vi "Lockin_sweep.vi"(0 "Transport":refnum<class "Transport.lvclass">, 3 "error in (no error)":errorcluster) -> (7 "Transport out":refnum<class "Transport.lvclass">, 10 "error out":errorcluster)   [LabVIEW 2019, in "Transport.lvclass"]
uses:
  Transport.lvclass
  Control Experiment/Control Experiment.lvclass
  <userlib>/LevyLab/Lockin-Multichannel/Instrument.DAQ/Typedefs/Sweep.Configuration--Cluster.ctl
  <userlib>/LevyLab/Lockin-Multichannel/Instrument.DAQ/Instrument.DAQ.lvclass
  <userlib>/LevyLab/Lockin-Multichannel/Instrument.DAQ/Typedefs/Sweep.Channel--Cluster.ctl
  <userlib>/LevyLab/Lockin-Multichannel/Instrument.Lockin/Instrument.Lockin.lvclass
  <userlib>/LevyLab/Lockin-Multichannel/Instrument.Lockin/Typedefs/Results Type--Enum.ctl
  <userlib>/LevyLab/Lockin-Multichannel/Instrument.DAQ/Typedefs/Sweep.Pattern--Enum.ctl
  <userlib>/LevyLab/Lockin-Multichannel/Instrument.DAQ/Typedefs/Sweep.Channel--Cluster--Array.ctl
  <vilib>/PRIrvin/XY Utilities/xy_utilities.lvlib
  217905a9-ad64-4e54-8703-31da4ffbd4c0.vi
  9896b5e5-a649-4b1b-acc0-fd49b17a1bc1.vi
  Typedefs/Lockin_Sweep JSON--Cluster.ctl
  <userlib>/LevyLab/Instrument Framework/Instrument Types/Cryostat/Typedefs/Magnet Axis--Enum.ctl
  <userlib>/LevyLab/Instrument Framework/Instrument Types/Cryostat/Instrument.Cryostat.lvclass
  <userlib>/LevyLab/Instrument Framework/Instrument Types/CBridge/Instrument.CBridge.lvclass
  <userlib>/LevyLab/Instrument Framework/Instrument Types/Strain/Instrument.Strain.lvclass
  C:/Program Files/National Instruments/LabVIEW 2019/user.lib/LevyLab/Instrument Framework/Instrument/Instrument.lvclass
  C:/Program Files/National Instruments/LabVIEW 2019/vi.lib/JKI/JKI SMO/SMO/SMO.lvclass
  <vilib>/PRIrvin/XY Utilities/subVIs/Divide float (multiple).vi
  <vilib>/PRIrvin/XY Utilities/subVIs/Multiply float (multiple).vi
  <vilib>/Utility/Data Type/NI_Data Type.lvlib
  <userlib>/LevyLab/Instrument Framework/Instrument/Instrument.lvclass
  <userlib>/LevyLab/Instrument Framework/Instrument Types/Lockin/Instrument.LockinAPI.lvclass
  <userlib>/LevyLab/Instrument Framework/Instrument Types/Amplifier/Instrument.Amplifier.lvclass
  <userlib>/LevyLab/Instrument Framework/Instrument Types/Delay Line/Instrument.DelayLine.lvclass
  <userlib>/LevyLab/Instrument Framework/Instrument Types/VNA/Instrument.VNA.lvclass
  <userlib>/LevyLab/Instrument Framework/Instrument Types/VSource/Instrument.VSource.lvclass
  Control Experiment/Typedefs/Instrument Types--enum.ctl
  Attributes/Instrument Attributes.lvlib
  ac72d6f7-f5c3-431a-8621-5120436d0f52.vi
  C:/Program Files/National Instruments/LabVIEW 2019/user.lib/LevyLab/Instrument Framework/Instrument Types/Lockin/Instrument.LockinAPI.lvclass
panel:
  in  "Start":bool
  in  "stop":bool
  in  "Tab Control":T1(tab)
  out "state history":string
  in  "Sweep Tables":cluster{"Ch":i32, "Table":dbl[]}[](array[cluster]) {"Table" format="%#_3p"; "Ch" min=1 max=16}
  in  "Emergency Stop Visible?":bool
  out "elapsed time (s)":i32=231
  in  "Experiment Comments":string
  in  "Experiment Folder":string
  out "time b/w points (ms)":u32=1037
  in  "Sweep Channels":T2 {"Table" format="%#_1f"; "Channel" min=1 max=128; "Start" format="%#_6p"; "End" format="%#_6p"}
  in  "Sweep Time (s)":dbl
  in  "Initial Wait (s)":dbl
  in  "Return to Start":bool
  out "Instrument Status":string
  in  "Emergency Stop 1":bool caption="Emergency Stop"
  out "Lockin (X)":cluster{"Wavenumber":dbl[], "Data":dbl[]}[](graph)
  out "Lockin (Y)":cluster{"Wavenumber":dbl[], "Data":dbl[]}[](graph)
  in  "Units":enum16{"ohms & siemens", "h/e2 & e2/h"}(ring)
  out "Resistance":cluster{"X-array":dbl[], "Y-array":dbl[]}[](graph)
  out "Conductance":cluster{"X-array":dbl[], "Y-array":dbl[]}[](graph)
  in  "Emergency Stop 2":bool caption="Emergency Stop"
  out "AI":cluster{"Wavenumber":dbl[], "Data":dbl[]}[](graph)
  out "AO":cluster{"Wavenumber":dbl[], "Data":dbl[]}[](graph)
  in  "Emergency Stop 3":bool caption="Emergency Stop"
  out "2 Terminal":cluster{"Wavenumber":dbl[], "Data":dbl[]}[](graph)
  out "4 Terminal":cluster{"Wavenumber":dbl[], "Data":dbl[]}[](graph)
  in  "Emergency Stop 4":bool caption="Emergency Stop"
  # "Configuration"
  # "Status"
  # "Metadata"
  # "VI Description"
  # "This VI uses the Lockin Sweep Method. That is, you tell the lockin to sweep from Start to End in a certain amount of time. The lockin will run independently while it executes the sweep. While the lockin is sweeping, this VI will poll the lockin once per second to get a snapshot of current results and the sweep status (sweeping or not sweeping). When the lockin is finished sweeping this VI will ask for the final sweep results and save them. The spacing between points is determined by the \"Fs Output\" control in the Lockin."
  # "*** These controls are only read if this VI is the top level. If is is called from Sweep Control then the folder and comments come from Sweep Control.vi ***"
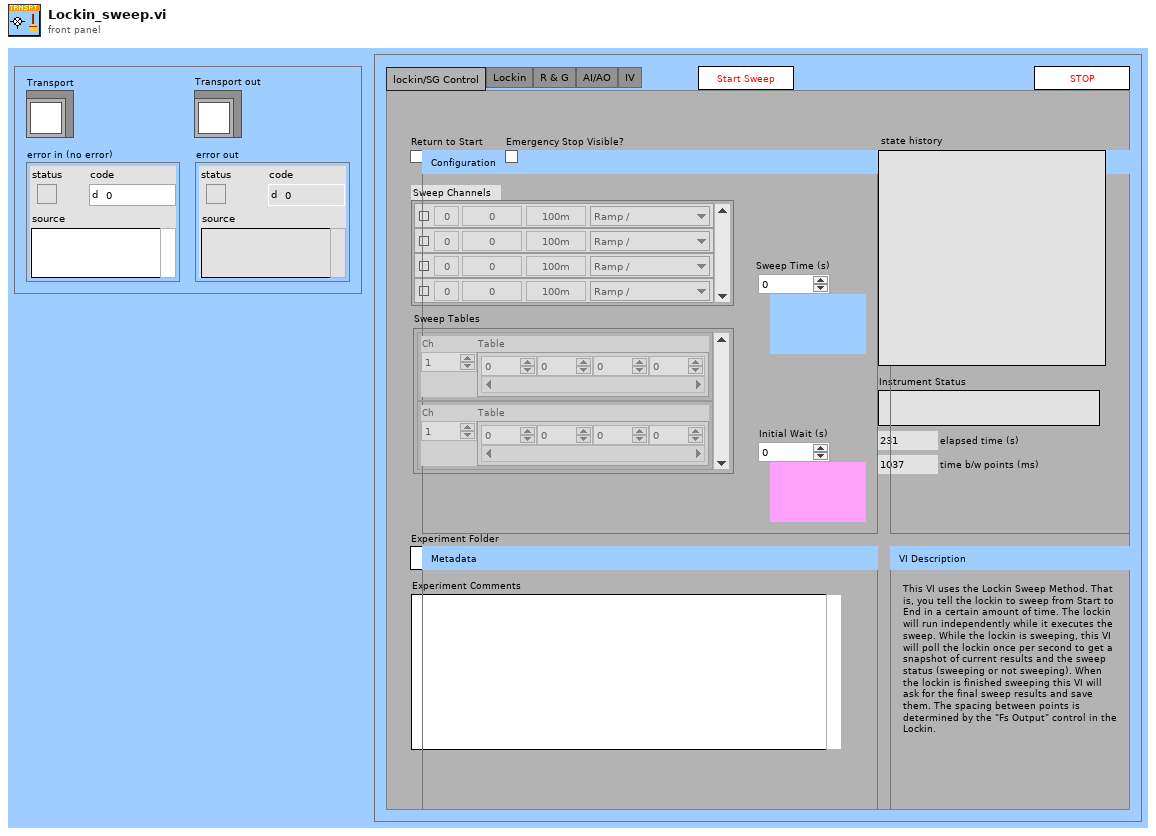
[diagram p1: front panel]
types:
  T1 = enum32{"lockin/SG Control", "Lockin", "R & G", "AI/AO", "IV"}
  T2 = typedef "Instrument.Lockin.lvlib/Instrument.DAQ.lvclass/Sweep.Channel--Cluster--Array.ctl" = T3[]
  T3 = typedef "Instrument.Lockin.lvlib/Instrument.DAQ.lvclass/Sweep.Channel--Cluster.ctl" = cluster{"Enable?":bool, "Channel":u16, "Start":dbl, "End":dbl, "Pattern":T4, "Table":dbl[]}
  T4 = typedef "Instrument.Lockin.lvlib/Instrument.DAQ.lvclass/Sweep.Pattern--Enum.ctl" = enum16{"Ramp /", "Ramp /\\", "Smooth Ramp _/", "Smooth Ramp _/\\_", "Table"}
  T5 = enum32{"Invalid", "Standard", "Closed", "Hidden", "Minimized", "Maximized"}
  T6 = enum32{"invalid app kind", "Development System", "Run Time System", "Student Edition", "Embedded LabVIEW", "Evaluation", "Custom"}
  T7 = enum32{"Bad", "Idle", "Run top level", "Running"}
  T8 = typedef "Control Experiment.lvclass/Instrument Types--enum.ctl" = enum16{"DAQ", "Amplifier", "Temperature", "Magnet", "Rotator", "Level", "Capacitance", "Delay Line", "Strain Cell", "VNA", "Source"}
  T9 = typedef "Instrument.Lockin.lvlib/Instrument.Lockin.lvclass/Results Type--Enum.ctl" = enum16{"X", "Y", "R", "Theta", "Mean"}
  T10 = typedef "Instrument.Lockin.lvlib/Instrument.DAQ.lvclass/Sweep.Configuration--Cluster.ctl" = cluster{"Sweep Time (s)":dbl, "Initial Wait (s)":dbl, "Return to Start":bool, "Channels":T2}
  T11 = typedef "Instrument.Cryostat.lvclass/Magnet Axis--Enum.ctl" = enum16{"X", "Y", "Z"}
  T12 = typedef "Transport.lvclass/Lockin_Sweep JSON--Cluster.ctl" = cluster{"Sweep Time (s)":dbl, "Initial Wait (s)":dbl, "Return to Start":bool, "Sweep Channels":T2, "Sweep Tables":cluster{"Ch":i32, "Table":dbl[]}[]}
  T13 = typedef "Control Experiment.lvclass/Instrument Classes--cluster.ctl" = cluster{"DAQ":refnum<class "Instrument.LockinAPI.lvclass">, "Amplifier":refnum<class "Instrument.Amplifier.lvclass">, "Temperature":refnum<class "Instrument.Cryostat.lvclass">, "Magnet":refnum<class "Instrument.Cryostat.lvclass">, "Rotator":refnum<class "Instrument.Cryostat.lvclass">, "Level":refnum<class "Instrument.Cryostat.lvclass">, "Capacitance":refnum<class "Instrument.CBridge.lvclass">, "Delay Line":refnum<class "Instrument.DelayLine.lvclass">, "Strain Cell":refnum<class "Instrument.Strain.lvclass">, "VNA":refnum<class "Instrument.VNA.lvclass">, "Source":refnum<class "Instrument.VSource.lvclass">}
  T14 = cluster{"Core":cluster{"Current VI Reference":refnum<vi>, "Close Panel on Exit?":bool}, "Transport":refnum<class "Transport.lvclass">, "C.E.":refnum<class "Control Experiment.lvclass">, "Instruments":T13, "Time":dbl, "Temperature":dbl, "Magnet":dbl, "Results (Dictionary)":cluster{"key":string, "value":dbl}[], "Sweep Value":dbl, "ms [0]":u32, "ms [i]":u32, "Execution:State":enum32{"Bad", "Idle", "Run top level", "Running"}, "Run Time System?":bool, "AO Waveforrm":waveform(dbl)[], "AI Waveform":waveform(dbl)[], "Sweep_AO":waveform(dbl)[], "Sweep_AI":waveform(dbl)[], "Sweep_X":waveform(dbl)[], "Sweep_Y":waveform(dbl)[], "Amplitude":dbl[], "UI stop":bool}
  T15 = cluster{"Current VI Reference":refnum<vi>, "Close Panel on Exit?":bool}
  T16 = cluster{"I-":i32, "I+":i32, "V1-":i32, "V1+":i32, "I2-":i32, "I2+":i32, "V2-":i32, "V2+":i32}
  T17 = typedef "Instrument.LockinAPI.lvclass/LockinAPI.getState.states--enum.ctl" = enum16{"idle", "created", "started", "stopped", "sweeping"}
  T18 = typedef "Instrument.Lockin.lvlib/Instrument.DAQ.lvclass/AO.Channel--Cluster--Array.ctl" = T19[]
  T19 = typedef "Instrument.Lockin.lvlib/Instrument.DAQ.lvclass/AO.Channel--Cluster.ctl" = cluster{"Enable?":bool, "Channel":i32, "Amplitude":dbl, "Offset":dbl, "Frequency":dbl, "Phase":dbl, "Function":T20, "Sweeping?":bool, "Limit AC":bool, "Limit DC?":bool, "Duty Cycle":bool}
  T20 = typedef "Instrument.Lockin.lvlib/Instrument.DAQ.lvclass/AO.Channel.Function--Enum.ctl" = enum16{"sine", "square", "triangle", "saw"}
  T21 = typedef "Instrument.LockinAPI.lvclass/LockinAPI.SweepData--Cluster.ctl" = cluster{"AO":waveform(dbl)[], "AI":waveform(dbl)[], "X":waveform(dbl)[], "Y":waveform(dbl)[]}
  T22 = typedef "LV-Data.lvclass/Dictionary--cluster.ctl" = cluster{"key":string, "value":variant}
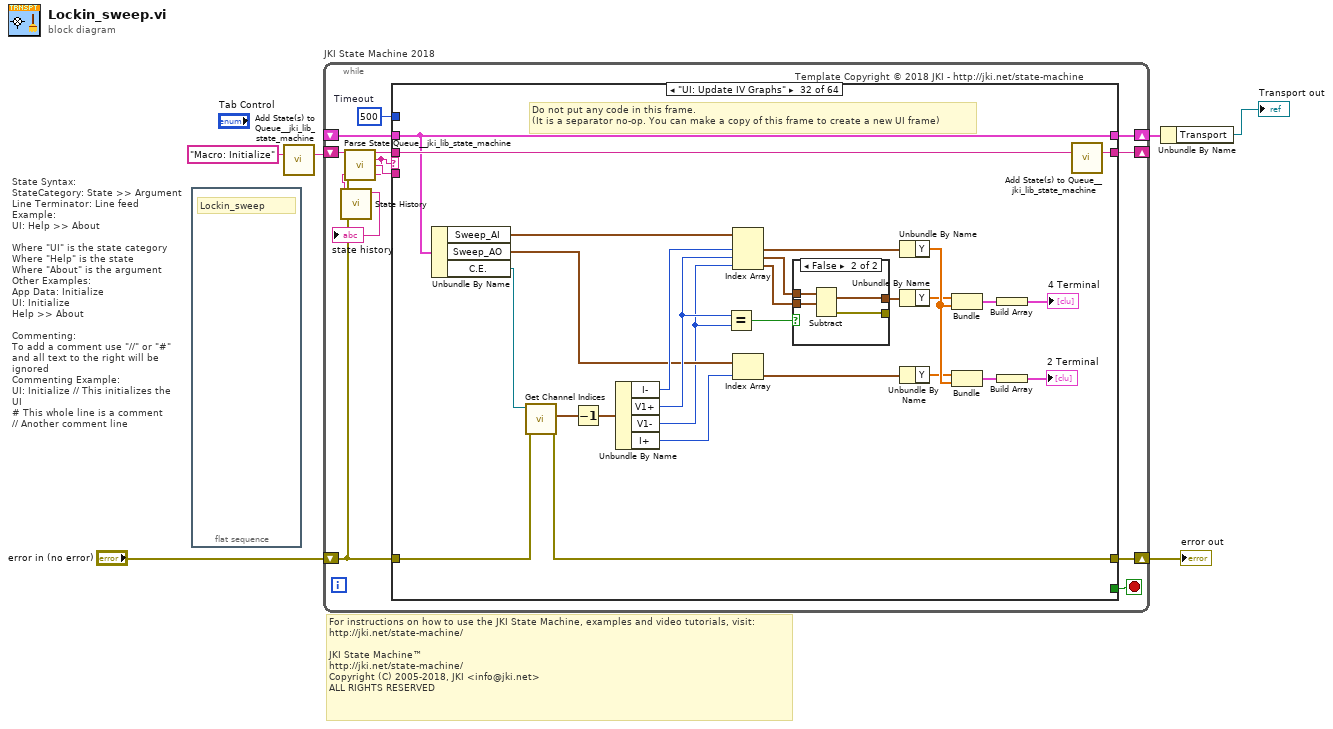
[diagram p0: block diagram]
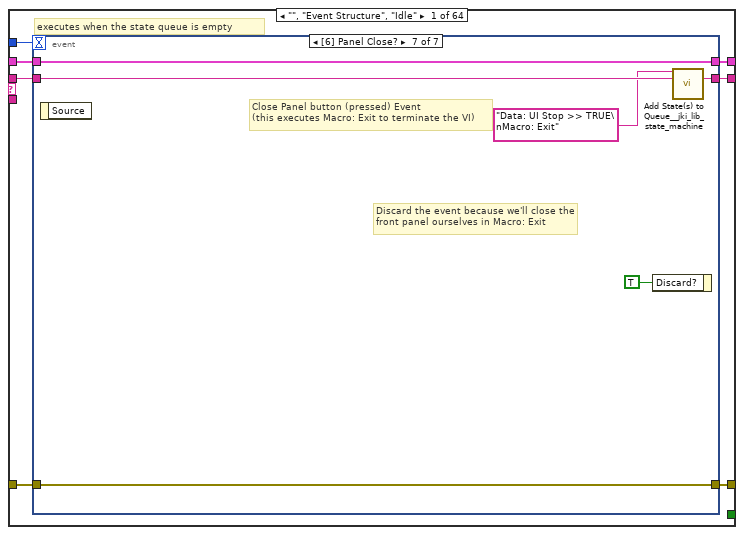
[diagram p2: hidden frame]
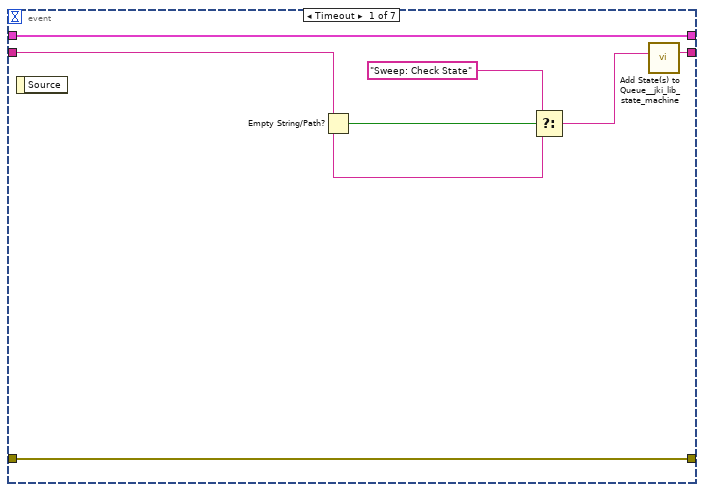
[diagram p3: hidden frame]
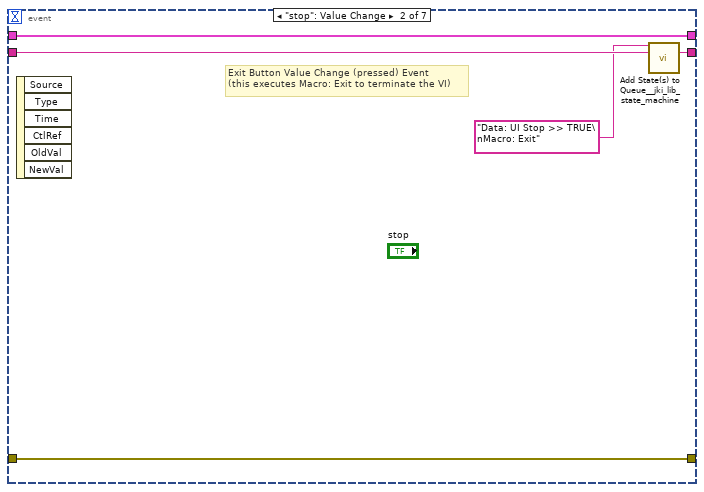
[diagram p4: hidden frame]
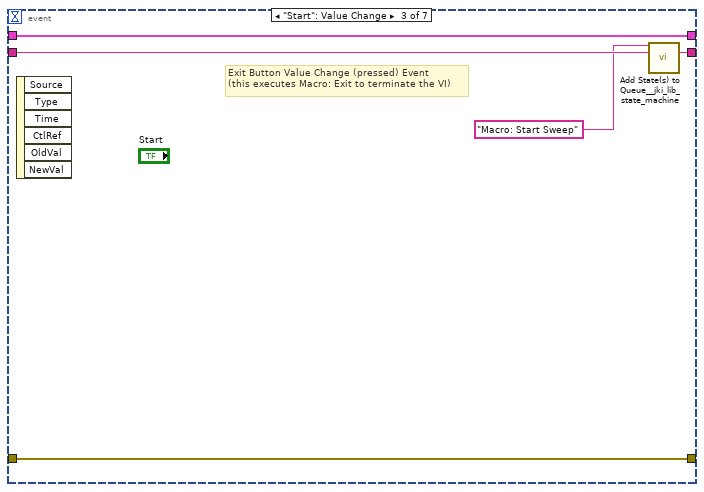
[diagram p5: hidden frame]
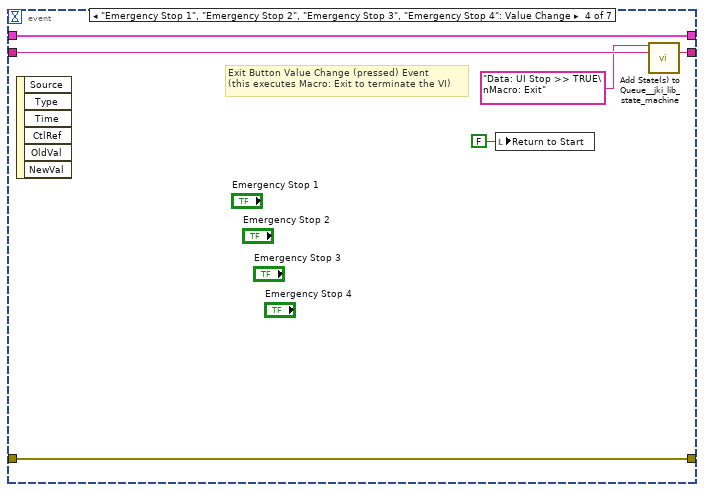
[diagram p6: hidden frame]
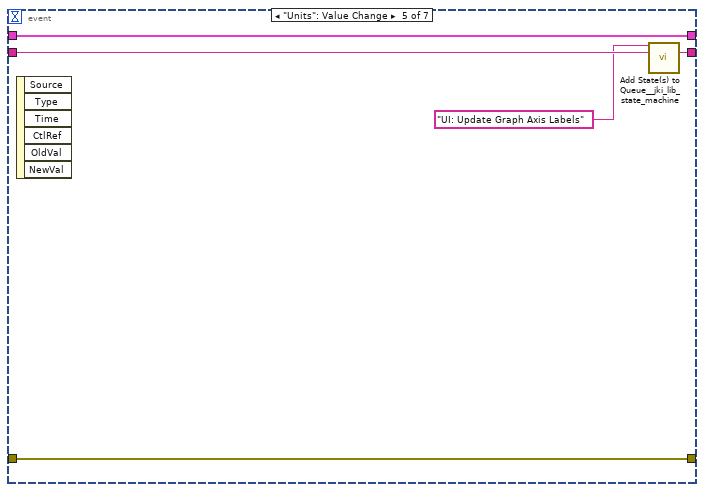
[diagram p7: hidden frame]
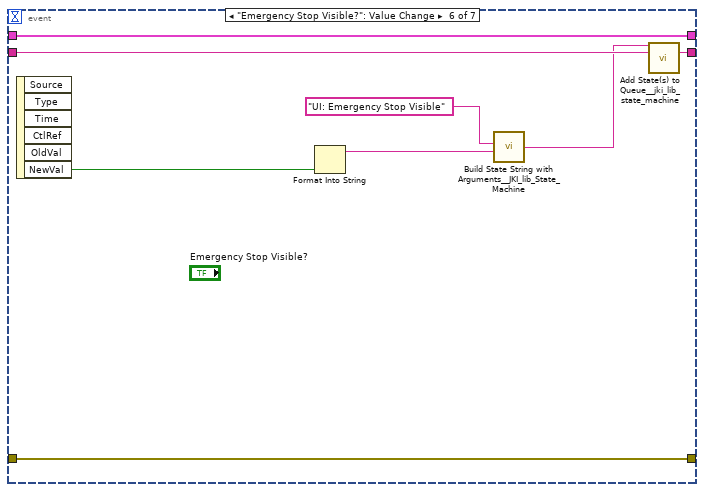
[diagram p8: hidden frame]
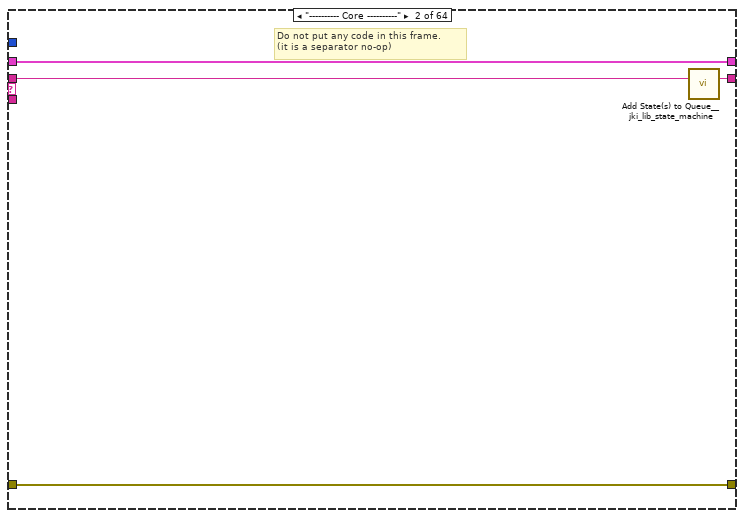
[diagram p9: hidden frame]
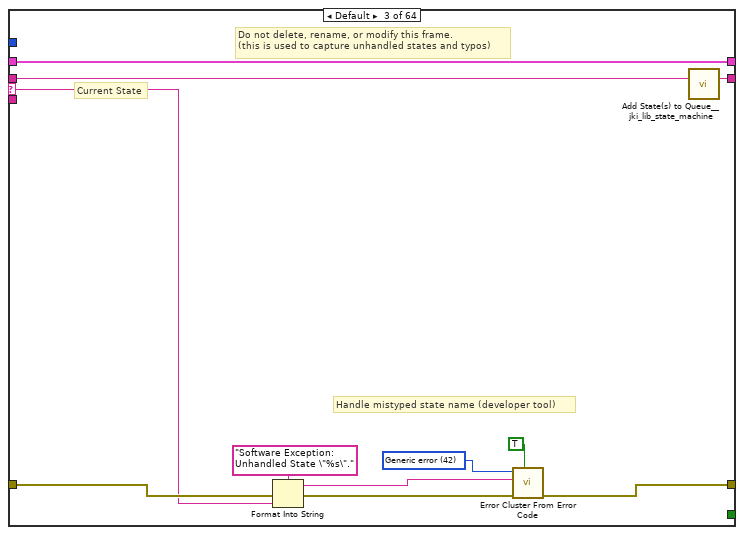
[diagram p10: hidden frame]
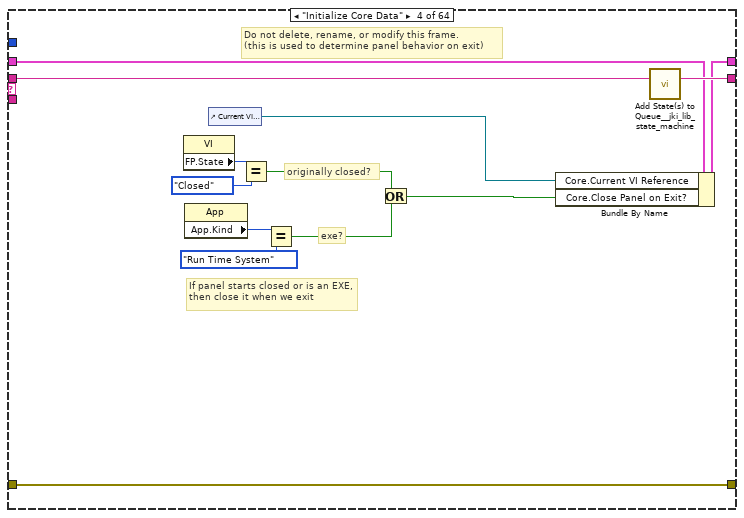
[diagram p11: hidden frame]
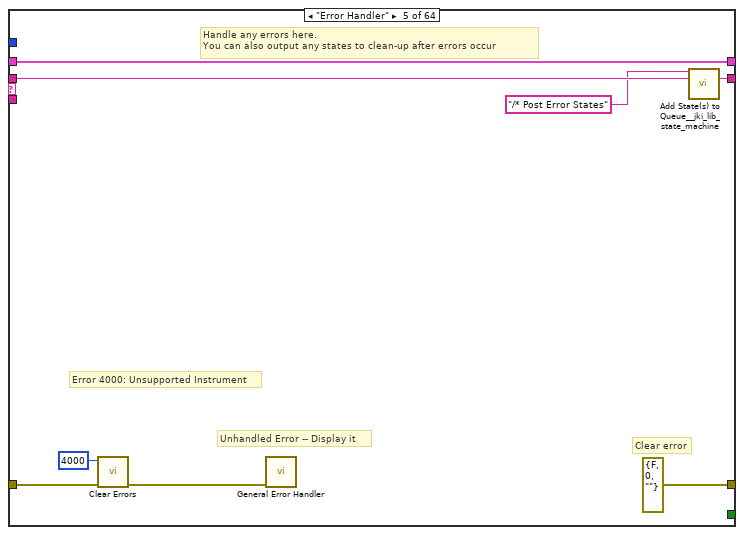
[diagram p12: hidden frame]
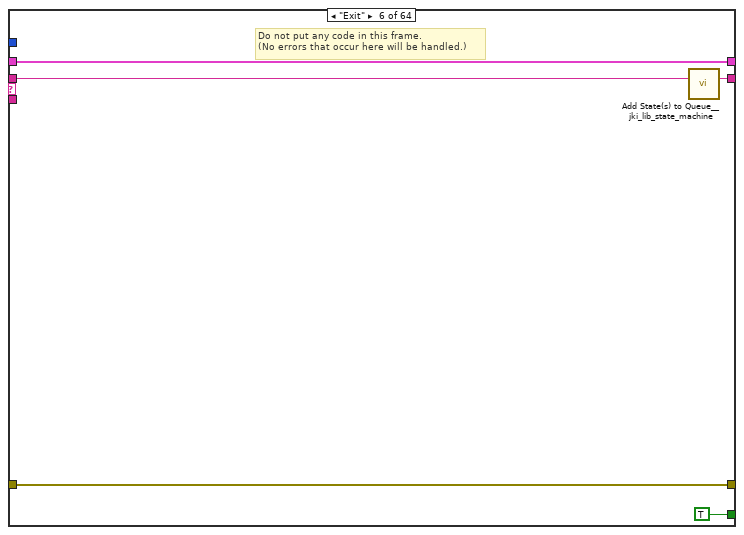
[diagram p13: hidden frame]
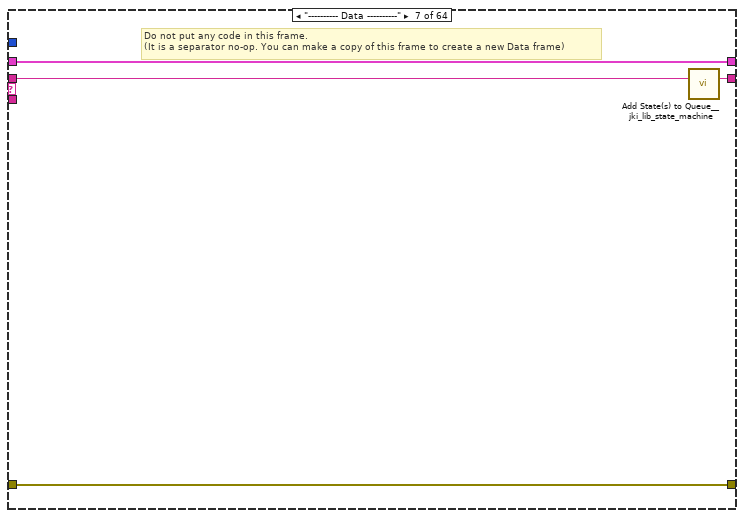
[diagram p14: hidden frame]
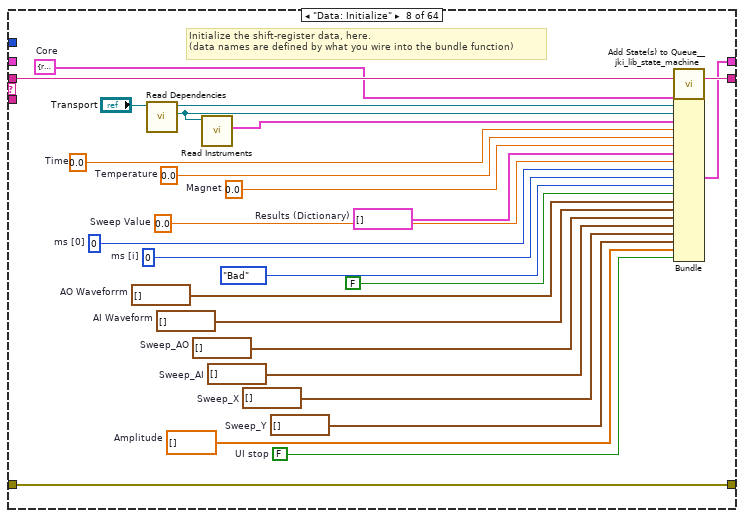
[diagram p15: hidden frame]
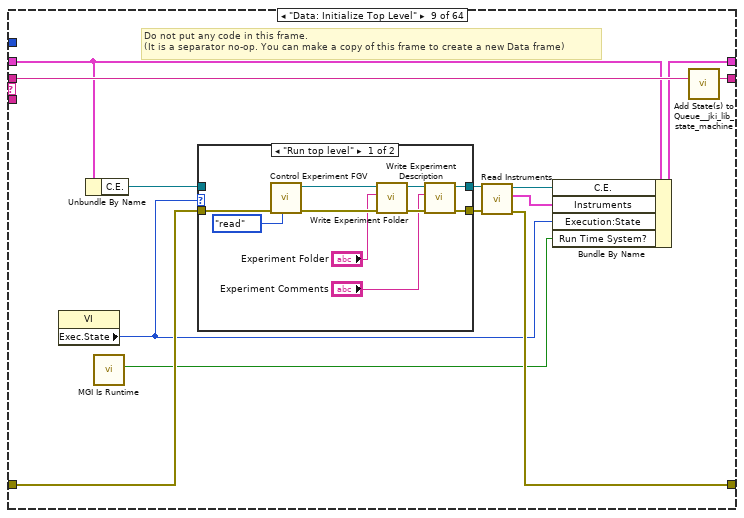
[diagram p16: hidden frame]
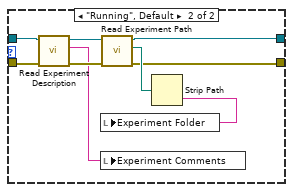
[diagram p17: hidden frame]
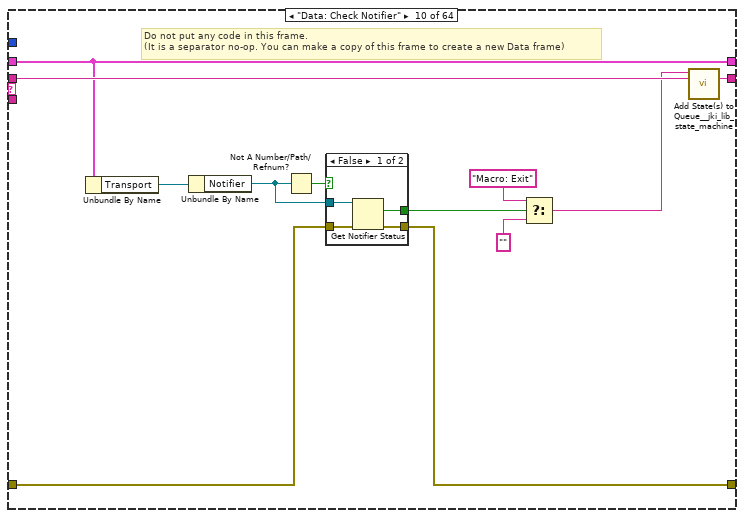
[diagram p18: hidden frame]
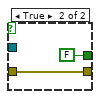
[diagram p19: hidden frame]
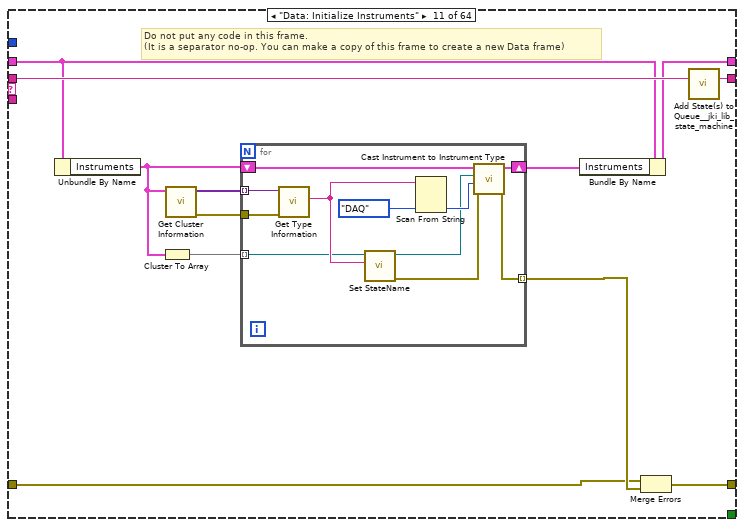
[diagram p20: hidden frame]
diagram:
  # "For instructions on how to use the JKI State Machine, examples and video tutorials, visit:\nhttp://jki.net/state-machine/\n\nJKI State Machine™\nhttp://jki.net/state-machine/\nCopyright (C) 2005-2018, JKI <info@jki.net>\nALL RIGHTS RESERVED"
  # "State Syntax:\nStateCategory: State >> Argument\nLine Terminator: Line feed\nExample:\nUI: Help >> About\n\nWhere \"UI\" is the state category\nWhere \"Help\" is the state\nWhere \"About\" is the argument\nOther Examples:\nApp Data: Initialize\nUI: Initialize\nHelp >> About\n\nCommenting:\nTo add a comment use \"//\" or \"#\" and all text to the right will be ignored\nCommenting Example:\nUI: Initialize // This initializes the UI\n# This whole line is a comment\n// Another comment line"
  n1 = flat-sequence {
    frame #0 {
      # "Lockin_sweep"
    }
  }
  n2 = call <vilib>:"Add State(s) to Queue__jki_lib_state_machine.vi"("State(s) in (\"\")"="Macro: Initialize") -> ("States Out"=w6:string)  [unwired: 14 in]
  n3 = while "JKI State Machine 2018" {
    shift-right: [w13] -> w4
    shift-left: _ -> [w12]
    shift-right: [w16] -> w2
    shift-left: "error in (no error)" -> [w10]
    shift-right: [w15] -> _
    shift-left: w6 -> [w9]
    stop <- w14 stop-if-true
    w11 = 500  # Timeout
    # "Template Copyright © 2018 JKI - http://jki.net/state-machine"
    n4 = call <vilib>:"Parse State Queue__jki_lib_state_machine.vi"("State Queue"=w9, "Error In (no error)"=w10) -> ("Remaining States"=w18:string, "Current State"=w8:string, "Arguments"=w17:string)  [unwired: 11 in]
    n5 = call "State History.vi"("Current State"=w8) -> ("History"=→"state history":string)  [unwired: 10 in]
    n6 = case shown="\"UI: Update IV Graphs\"" w8 {
      selector: w8 -> [_ _ w72 _ _ _ _ _ _ _ _ _ _ _ _ _ _ _ _ _ _ _ _ _ _ _ _ _ _ _ _ _ _ _ _ _ _ _ _ _ _ _ _ _ _ _ _ _ _ _ _ _ _ _ _ _ _ _ _ _ _ _ _ _]
      tunnel: w18 -> [w25 w71 w76 w95 w103 w108 w112 w138 w151 w182 w200 w224 w255 w290 w302 w329 w347 w359 w370 w376 w387 w403 w418 w444 w461 w481 w519 w568 w593 w608 w626 w673 w685 w754 w764 w769 w782 w795 w800 w812 w823 w827 w860 w886 w898 w912 w936 w949 w953 w957 w968 w983 w1005 w1033 w1066 w1088 w1110 w1132 w1164 w1185 w1189 w1193 w1213 w1232]
      tunnel: w17 -> [_ _ _ _ _ _ _ _ _ _ _ _ _ _ _ w324 _ _ _ w371 w383 _ w405 _ _ _ _ w562 w582 _ _ _ w679 _ _ _ _ _ _ _ _ _ _ _ _ _ _ _ _ _ _ _ _ _ _ _ _ _ _ _ _ _ _ _]
      tunnel: w12 -> [w23 w68 w74 w88 w100 w106 w109 _ w141 w180 w197 w221 w252 w275 w296 w325 w339 w356 w361 w374 w384 w399 w415 w434 w457 w478 w516 w566 w585 w600 w623 w663 w681 w751 w757 w766 w778 w791 w796 w804 w820 w824 w857 w884 w892 w910 w934 w946 w951 w954 w961 w977 w998 w1024 w1060 w1082 w1104 w1126 w1156 w1183 w1186 w1190 w1201 w1227]
      tunnel: [w22 w69 w78 w92 errorcluster {"status"=FALSE, "code"=0, "source"=""} ("error out") w105 w110 w135 w143 w173 w196 w214 w251 w277 w294 w327 w340 w357 w363 w372 w385 w395 w416 w439 w459 w479 w517 w565 w586 w606 w624 w654 w682 w752 w762 w767 w771 w793 w798 w810 w821 w825 w828 w879 w896 w905 w923 w947 w950 w955 w959 w971 w993 w1022 w1053 w1076 w1098 w1120 w1162 w1180 w1187 w1191 w1204 w1225] -> w16
      tunnel: w10 -> [w21 w69 w77 w92 w97 w105 w110 w135 w144 w172 w189 w215 w250 w284 w297 w327 w331 w357 w368 w373 w385 w390 w416 w438 w455 w470 w503 w565 w580 w606 w624 w655 w683 w752 w762 w767 w770 w793 w798 w810 w821 w825 w834 w875 w887 w901 w913 w947 w950 w955 w960 w981 w1000 w1020 w1061 w1083 w1105 w1127 w1140 w1171 w1187 w1191 w1196 w1220]
      tunnel: [w24 w70 w75 w94 w102 w107 w111 w137 w150 w181 w199 w223 w254 w289 w301 w328 w346 w358 w369 w375 w386 w402 w417 w443 w460 w480 w518 w567 w592 w607 w625 w672 w684 w753 w763 w768 w781 w794 w799 w811 w822 w826 w859 w885 w897 w911 w935 w948 w952 w956 w967 w982 w1004 w1032 w1065 w1087 w1109 w1131 w1163 w1184 w1188 w1192 w1212 w1231] -> w15
      tunnel: [_ _ _ _ _ TRUE _ _ _ _ _ _ _ _ _ _ _ _ _ _ _ _ _ _ _ _ _ _ _ _ _ _ _ _ _ _ _ _ _ _ _ _ _ _ _ _ _ _ _ _ _ _ _ _ _ _ _ _ _ _ _ _ _ _] -> w14
      tunnel: [w20 w68 w74 w93 w100 w106 w109 w136 w142 w180 w198 w222 w253 w285 w295 w326 w343 w356 w364 w374 w384 w398 w415 w434 w457 w478 w516 w566 w585 w600 w623 w663 w681 w751 w757 w766 w778 w791 w796 w804 w820 w824 w858 w883 w893 w909 w933 w946 w951 w954 w965 w980 w1003 w1025 w1064 w1086 w1108 w1130 w1155 w1182 w1186 w1190 w1202 w1228] -> w13
      tunnel: w11 -> [w19 _ _ _ _ _ _ _ _ _ _ _ _ _ _ _ _ _ _ _ _ _ _ _ _ _ _ _ _ _ _ _ _ _ _ _ _ _ _ _ _ _ _ _ _ _ _ _ _ _ _ _ _ _ _ _ _ _ _ _ _ _ _ _]
      frame "", "Event Structure", "Idle" {
        # "executes when the state queue is empty"
        n7 = event shown="[6] Panel Close?" {
          selector: _ -> [_ _ _ _ _ _ _]
          dyn-events: _ -> [_ _ _ _ _ _ _]
          timeout: w19 -> [_ _ _ _ _ _ _]
          tunnel: w25 -> [w27 w37 w42 w48 w53 w61 w67]
          tunnel: [w32 w36 w41 w47 w52 w60 w66] -> w24
          tunnel: w23 -> [w30 w33 w38 w45 w50 w58 w64]
          tunnel: [w31 w35 w40 w46 w51 w59 w65] -> w22
          tunnel: w21 -> [w31 w35 w40 w46 w51 w59 w65]
          tunnel: [w30 w33 w38 w45 w50 w58 w64] -> w20
          event Timeout {
            n8 = event-data() -> ()  [unwired: 1 in, 1 out]
            n9 = Empty String/Path?(string/path=w27) -> (empty?=w29:bool)
            n10 = Select(t="Sweep: Check State" ("State(s) in Front (\"\")"), s=w29, f=w27) -> (s? t:f=w28:string)
            n11 = call <vilib>:"Add State(s) to Queue__jki_lib_state_machine.vi"("State(s) in (\"\")"=w28) -> ("States Out"=w32:string)  [unwired: 14 in]
          }
          event "stop": Value Change {
            # "Exit Button Value Change (pressed) Event\n(this executes Macro: Exit to terminate the VI)"
            n12 = event-data() -> ()  [unwired: 1 in, 6 out]
            n13 = call <vilib>:"Add State(s) to Queue__jki_lib_state_machine.vi"("State(s) in Front (\"\")"="Data: UI Stop >> TRUE\nMacro: Exit", "State(s) in (\"\")"=w37) -> ("States Out"=w36:string)  [unwired: 13 in]
          }
          event "Start": Value Change {
            # "Exit Button Value Change (pressed) Event\n(this executes Macro: Exit to terminate the VI)"
            n14 = event-data() -> ()  [unwired: 1 in, 6 out]
            n15 = call <vilib>:"Add State(s) to Queue__jki_lib_state_machine.vi"("State(s) in Front (\"\")"="Macro: Start Sweep", "State(s) in (\"\")"=w42) -> ("States Out"=w41:string)  [unwired: 13 in]
          }
          event "Emergency Stop 1", "Emergency Stop 2", "Emergency Stop 3", "Emergency Stop 4": Value Change {
            # "Exit Button Value Change (pressed) Event\n(this executes Macro: Exit to terminate the VI)"
            n16 = event-data() -> ()  [unwired: 1 in, 6 out]
            n17 = local write "Return to Start"(FALSE ("Return to Start")) -> ()
            n18 = call <vilib>:"Add State(s) to Queue__jki_lib_state_machine.vi"("State(s) in Front (\"\")"="Data: UI Stop >> TRUE\nMacro: Exit", "State(s) in (\"\")"=w48) -> ("States Out"=w47:string)  [unwired: 13 in]
          }
          event "Units": Value Change {
            n19 = event-data() -> ()  [unwired: 1 in, 6 out]
            n20 = call <vilib>:"Add State(s) to Queue__jki_lib_state_machine.vi"("State(s) in Front (\"\")"="UI: Update Graph Axis Labels", "State(s) in (\"\")"=w53) -> ("States Out"=w52:string)  [unwired: 13 in]
          }
          event "Emergency Stop Visible?": Value Change {
            n21 = event-data() -> ("NewVal"=w55:bool)  [unwired: 1 in, 5 out]
            n22 = Format Into String(w55) -> (resulting string=w57:string)  [unwired: 3 in, 1 out]
            n23 = call <vilib>:"Build State String with Arguments__JKI_lib_State_Machine.vi"("Arguments (\"\")"=w57, "State"="UI: Emergency Stop Visible") -> ("State with Arguments"=w54:string)  [unwired: 4 in]
            n24 = call <vilib>:"Add State(s) to Queue__jki_lib_state_machine.vi"("State(s) in Front (\"\")"=w54, "State(s) in (\"\")"=w61) -> ("States Out"=w60:string)  [unwired: 13 in]
          }
          event Panel Close? {
            # "Discard the event because we'll close the front panel ourselves in Macro: Exit"
            # "Close Panel button (pressed) Event\n(this executes Macro: Exit to terminate the VI)"
            n25 = event-data() -> ()  [unwired: 1 in, 1 out]
            n26 = event-data("Discard?"=TRUE) -> ()  [unwired: 1 in, 1 out]
            n27 = call <vilib>:"Add State(s) to Queue__jki_lib_state_machine.vi"("State(s) in Front (\"\")"="Data: UI Stop >> TRUE\nMacro: Exit", "State(s) in (\"\")"=w67) -> ("States Out"=w66:string)  [unwired: 13 in]
          }
        }
      }
      frame "---------- Core ----------" {
        # "Do not put any code in this frame.\n(it is a separator no-op)"
        n28 = call <vilib>:"Add State(s) to Queue__jki_lib_state_machine.vi"("State(s) in (\"\")"=w71) -> ("States Out"=w70:string)  [unwired: 14 in]
      }
      frame Default {
        w81 = 42 items=["No error", "Argument error", "Memory is full", "Out of zone", "End of file", "File already open", "Generic file I/O error", "File not found", "File permission error", "Disk is full", "Duplicate path", "Too many files open", "System feature not enabled", "Resource file not found", "Cannot add resource", "Resource not found", "Image not found", "Image memory error", "Pen does not exist", "Config type invalid", "Config token not found", "Config parse error", "Config memory error", "Bad external code format", "Bad external code offset", "External code not present", "Null window", "Destroy window error", "Null menu", "Print aborted", "Bad print record", "Print driver error", "Windows error during printing", "Memory error during printing", "Print dialog error", "Generic print error", "Invalid device refnum", "Device not found", "Device parameter error", "Device unit error", "Cannot open device", "Device call aborted", "Generic error", "Cancelled by user", "Object ID too low", "Object ID too high", "Object not in heap", "Unknown heap", "Unknown object (invalid DefProc)", "Unknown object (DefProc not in table)", "Message out of range", "Invalid (null) method", "Unknown message", "Manager call not supported", "Bad address", "Network operation in progress", "Network operation timed out", "Connection is busy", "Network attribute not supported", "Network error", "Address in use", "System out of memory", "Connection aborted", "Connection refused", "Not connected", "Already connected", "Connection closed", "Initialization error (interapplication manager)", "Bad occurrence", "Wait on unbound occurrence handler", "Occurrence queue overflow", "Datalog type conflict", "Unused", "Unrecognized type (interapplication manager)", "Memory corrupt", "Failed to make temporary DLL", "Old CIN version", "Drag socket not found", "Failed to load drop-object", "Failed to register OLE object", "Failed to release OLE object", "Format specifier type mismatch", "Unknown format specifier", "Too few format specifiers", "Too many format specifiers", "Scan failed", "Newer CIN version", "Error converting to variant", "Runtime menu error", "Password tampered", "Variant attribute not found", "Incompatible variant data type", "Event data is not available", "Event Store is not present", "Occurrence is not found", "Event Queue is not created", "Event info is not available", "Refnum passed is NULL", "Error retrieving Class GUID", "Error retrieving CoClass GUID", "Error retrieving TypeLib GUID.", "Bad built application magic bytes.", "Specific driver is different from the specific driver associated with the Logical Name.", "There is no session opened to the class driver.", "Max Error", "MAX - Error with config objects", "MAX - Error loading configuration", "MAX - Group not supported"]
        # "Current State"
        # "Do not delete, rename, or modify this frame.\n(this is used to capture unhandled states and typos)"
        # "Handle mistyped state name (developer tool)"
        n29 = Format Into String(format string="Software Exception: Unhandled State \"%s\"." ("message"), error in=w77, w72) -> (resulting string=w80:string, error out=w79:errorcluster)  [unwired: 1 in]
        n30 = call <vilib>:"Error Cluster From Error Code.vi"("show call chain? (False)"=TRUE, "error in (no error)"=w79, "error message (\"\")"=w80, "error code (0)"=w81) -> ("error out"=w78:errorcluster)  [unwired: 5 in]
        n31 = call <vilib>:"Add State(s) to Queue__jki_lib_state_machine.vi"("State(s) in (\"\")"=w76) -> ("States Out"=w75:string)  [unwired: 14 in]
      }
      frame "Initialize Core Data" {
        # "Do not delete, rename, or modify this frame.\n(this is used to determine panel behavior on exit)"
        # "originally closed?"
        # "exe?"
        # "If panel starts closed or is an EXE, then close it when we exit"
        n32 = property class="VI"() -> ("FP.State"=w85:T5)  [unwired: 2 in, 2 out]
        n33 = property class="App"() -> ("App.Kind"=w91:T6)  [unwired: 2 in, 2 out]
        n34 = control-ref of="Current VI Reference"() -> (w86:refnum<vi>)
        n35 = Equal?(x=w85, y=T5."Closed" ("Front Panel Window:State")) -> (x = y?=w83:bool)
        n36 = Equal?(x=w91, y=T6."Run Time System" ("Application:Kind")) -> (x = y?=w89:bool)
        n37 = Or(x=w83, y=w89) -> (x .or. y?=w87:bool)
        n38 = Bundle By Name(cluster=w88, "Core.Current VI Reference"=w86, "Core.Close Panel on Exit?"=w87) -> (w93:T14)
        n39 = call <vilib>:"Add State(s) to Queue__jki_lib_state_machine.vi"("State(s) in (\"\")"=w95) -> ("States Out"=w94:string)  [unwired: 14 in]
      }
      frame "Error Handler" {
        # "Error 4000: Unsupported Instrument"
        # "Unhandled Error -- Display it"
        # "Handle any errors here.\nYou can also output any states to clean-up after errors occur"
        # "Clear error"
        n40 = call <vilib>:"Clear Errors.vi"("error in (no error)"=w97, "specific error code to clear (0: all)"=4000) -> ("error out"=w96:errorcluster)  [unwired: 4 in, 1 out]
        n41 = call <vilib>:"General Error Handler.vi"("error in (no error)"=w96) -> ()  [unwired: 10 in, 5 out]
        n42 = call <vilib>:"Add State(s) to Queue__jki_lib_state_machine.vi"("State(s) in Front (\"\")"="/* Post Error States", "State(s) in (\"\")"=w103) -> ("States Out"=w102:string)  [unwired: 13 in]
      }
      frame "Exit" {
        # "Do not put any code in this frame.\n(No errors that occur here will be handled.)"
        n43 = call <vilib>:"Add State(s) to Queue__jki_lib_state_machine.vi"("State(s) in (\"\")"=w108) -> ("States Out"=w107:string)  [unwired: 14 in]
      }
      frame "---------- Data ----------" {
        # "Do not put any code in this frame.\n(It is a separator no-op. You can make a copy of this frame to create a new Data frame)"
        n44 = call <vilib>:"Add State(s) to Queue__jki_lib_state_machine.vi"("State(s) in (\"\")"=w112) -> ("States Out"=w111:string)  [unwired: 14 in]
      }
      frame "Data: Initialize" {
        w115 = FALSE  # UI stop
        w118 = dbl[] []  # Amplitude
        w122 = waveform(dbl)[] []  # Sweep_Y
        w123 = waveform(dbl)[] []  # Sweep_X
        w119 = cluster{"key":string, "value":dbl}[] []  # Results (Dictionary)
        w125 = waveform(dbl)[] []  # Sweep_AO
        w124 = waveform(dbl)[] []  # Sweep_AI
        w126 = waveform(dbl)[] []  # AI Waveform
        w127 = waveform(dbl)[] []  # AO Waveforrm
        w128 = 0.0  # Sweep Value
        w129 = u32 0  # ms [i]
        w130 = u32 0  # ms [0]
        w132 = 0.0  # Time
        w133 = 0.0  # Magnet
        w131 = 0.0  # Temperature
        w134 = T15 {"Current VI Reference"=refnum, "Close Panel on Exit?"=FALSE}  # Core
        # "Initialize the shift-register data, here.\n(data names are defined by what you wire into the bundle function)"
        n45 = call "Read Dependencies.vi"("Transport"="Transport") -> ("C.E."=w117:refnum<class "Control Experiment.lvclass">, "Transport"=w120:refnum<class "Transport.lvclass">)  [unwired: 8 in, 1 out]
        n46 = call "Read Instruments.vi"("Control Experiment in"=w117) -> ("Instruments"=w116:T13)  [unwired: 8 in, 2 out]
        n47 = call <vilib>:"Add State(s) to Queue__jki_lib_state_machine.vi"("State(s) in (\"\")"=w138) -> ("States Out"=w137:string)  [unwired: 14 in]
        n48 = Bundle("Core"=w134, "Transport"=w120, "C.E."=w117, "Instruments"=w116, "Time"=w132, "Temperature"=w131, "Magnet"=w133, "Results (Dictionary)"=w119, "Sweep Value"=w128, "ms [0]"=w130, "ms [i]"=w129, "Execution:State"=T7."Bad", "Run Time System?"=FALSE, "AO Waveforrm"=w127, "AI Waveform"=w126, "Sweep_AO"=w125, "Sweep_AI"=w124, "Sweep_X"=w123, "Sweep_Y"=w122, "Amplitude"=w118, "UI stop"=w115) -> (w136:T14)  [unwired: 1 in]
      }
      frame "Data: Initialize Top Level" {
        # "Do not put any code in this frame.\n(It is a separator no-op. You can make a copy of this frame to create a new Data frame)"
        n49 = property class="VI"() -> ("Exec.State"=w140:T7)  [unwired: 2 in, 2 out]
        n50 = Unbundle By Name(w141) -> ("C.E."=w145:refnum<class "Control Experiment.lvclass">)
        n51 = call <userlib>:"MGI Is Runtime.vi"() -> ("Run Time System?"=w139:bool)  [unwired: 7 in]
        n52 = case shown="\"Run top level\"" w140 {
          tunnel: w144 -> [w161 w166]
          tunnel: [w156 w165] -> w146
          tunnel: [w155 w164] -> w147
          tunnel: w145 -> [_ w167]
          frame "Run top level" {
            n53 = call "Control Experiment FGV.vi"("Function"=enum16{"read", "write"}."read", "error in (no error)"=w161) -> ("error out"=w159:errorcluster, "Control Experiment.lvclass out"=w160:refnum<class "Control Experiment.lvclass">)  [unwired: 8 in]
            n54 = call "Write Experiment Folder.vi"("error in (no error)"=w159, "Experiment Folder"="Experiment Folder", "Control Experiment in"=w160) -> ("error out"=w157:errorcluster, "Control Experiment out"=w158:refnum<class "Control Experiment.lvclass">)  [unwired: 7 in]
            n55 = call "Write Experiment Description.vi"("error in (no error)"=w157, "Experiment Description"="Experiment Comments", "Control Experiment in"=w158) -> ("error out"=w156:errorcluster, "Control Experiment out"=w155:refnum<class "Control Experiment.lvclass">)  [unwired: 7 in]
          }
          frame "Running", Default {
            n56 = call "Read Experiment Description.vi"("error in (no error)"=w166, "Control Experiment in"=w167) -> ("error out"=w169:errorcluster, "Experiment Description"=w162:string, "Control Experiment out"=w168:refnum<class "Control Experiment.lvclass">)  [unwired: 7 in]
            n57 = local write "Experiment Comments"(w162) -> ()
            n58 = call "Read Experiment Path.vi"("error in (no error)"=w169, "Control Experiment in"=w168) -> ("error out"=w165:errorcluster, "Experiment Path"=w170:path, "Control Experiment out"=w164:refnum<class "Control Experiment.lvclass">)  [unwired: 7 in]
            n59 = Strip Path(path=w170) -> (name=w163:string)  [unwired: 1 out]
            n60 = local write "Experiment Folder"(w163) -> ()
          }
        }
        n61 = call "Read Instruments.vi"("error in (no error)"=w146, "Control Experiment in"=w147) -> ("error out"=w143:errorcluster, "Instruments"=w149:T13, "Control Experiment out"=w148:refnum<class "Control Experiment.lvclass">)  [unwired: 7 in]
        n62 = Bundle By Name(cluster=w141, "C.E."=w148, "Instruments"=w149, "Execution:State"=w140, "Run Time System?"=w139) -> (w142:T14)
        n63 = call <vilib>:"Add State(s) to Queue__jki_lib_state_machine.vi"("State(s) in (\"\")"=w151) -> ("States Out"=w150:string)  [unwired: 14 in]
      }
      frame "Data: Check Notifier" {
        # "Do not put any code in this frame.\n(It is a separator no-op. You can make a copy of this frame to create a new Data frame)"
        n64 = Unbundle By Name(w180) -> ("Transport"=w179:refnum<class "Transport.lvclass">)
        n65 = Unbundle By Name(w179) -> ("Notifier"=w171:refnum<notifier>)
        n66 = Not A Number/Path/Refnum?(number/path/refnum=w171) -> (NaN/Path/Refnum?=w178:bool)
        n67 = case shown="False" w178 {
          tunnel: [w186 FALSE] -> w177
          tunnel: [w185 w187] -> w173
          tunnel: w171 -> [w184 _]
          tunnel: w172 -> [w183 w187]
          frame False {
            n68 = Get Notifier Status(notifier=w184, error in (no error)=w183) -> (current notification=w186:bool, error out=w185:errorcluster)  [unwired: 3 out]
          }
          frame True {
          }
        }
        n69 = Select(t="Macro: Exit", s=w177, f="") -> (s? t:f=w174:string)
        n70 = call <vilib>:"Add State(s) to Queue__jki_lib_state_machine.vi"("State(s) in Front (\"\")"=w174, "State(s) in (\"\")"=w182) -> ("States Out"=w181:string)  [unwired: 13 in]
      }
      frame "Data: Initialize Instruments" {
        # "Do not put any code in this frame.\n(It is a separator no-op. You can make a copy of this frame to create a new Data frame)"
        n71 = Unbundle By Name(w197) -> ("Instruments"=w190:T13)
        n72 = Cluster To Array(cluster=w190) -> (array=w195:refnum<class "Instrument.lvclass">[])
        n73 = call <vilib>:"Get Cluster Information.vi"("variant"=w190) -> ("error out"=w193:errorcluster, "cluster elements"=w194:variant[])  [unwired: 9 in]
        n74 = for {
          tunnel: w195 -> [w201] mode=indexing
          tunnel: [w209] -> w192 mode=indexing
          shift-right: [w210] -> w191
          shift-left: w190 -> [w211]
          tunnel: w194 -> [w206] mode=indexing
          tunnel: w193 -> [w205]
          n75 = call <vilib>:"Get Type Information.vi"("error in (no error)"=w205, "variant"=w206) -> ("name"=w202:string)  [unwired: 5 in, 4 out]
          n76 = call "Set StateName.vi"("StateName"=w202, "SMO"=w201) -> ("error out"=w203:errorcluster, "SMO out"=w204:refnum<class "Instrument.lvclass">)  [unwired: 8 in]
          n77 = Scan From String(input string=w202, default 1=Instrument_Types--enum."DAQ" ("Type")) -> (output 1=w207:T8)  [unwired: 3 in, 3 out]
          n78 = call "Cast Instrument to Instrument Type.vi"("error in (no error)"=w203, "Type"=w207, "Instrument in"=w204, "Instrument Classes"=w211) -> ("error out"=w209:errorcluster, "Instrument Classes out"=w210:T13)  [unwired: 5 in, 1 out]
        }
        n79 = Bundle By Name(cluster=w197, "Instruments"=w191) -> (w198:T14)
        n80 = Merge Errors(w189, w192) -> (w196:errorcluster)
        n81 = call <vilib>:"Add State(s) to Queue__jki_lib_state_machine.vi"("State(s) in (\"\")"=w200) -> ("States Out"=w199:string)  [unwired: 14 in]
      }
      frame "Data: Disable Unsupported Instruments" {
        # "Do not put any code in this frame.\n(It is a separator no-op. You can make a copy of this frame to create a new Data frame)"
        n82 = Unbundle By Name(w221) -> ("Instruments"=w213:T13)
        n83 = call <vilib>:"Get Cluster Information.vi"("variant"=w213) -> ("error out"=w218:errorcluster, "cluster elements"=w219:variant[])  [unwired: 9 in]
        n84 = Cluster To Array(cluster=w213) -> (array=w220:refnum<class "Instrument.lvclass">[])
        n85 = for {
          tunnel: w220 -> [w231] mode=indexing
          tunnel: [w236] -> w217 mode=indexing
          shift-right: [w237] -> w212
          shift-left: w213 -> [w238]
          tunnel: w219 -> [w233] mode=indexing
          tunnel: w218 -> [w232]
          tunnel: string[] ["Lockin", "Amplifier", "Level", "VNA", "Source"] ("element") -> [w228]
          n86 = call <vilib>:"Get Type Information.vi"("error in (no error)"=w232, "variant"=w233) -> ("name"=w227:string)  [unwired: 5 in, 4 out]
          n87 = Search 1D Array(1D array=w228, element=w227) -> (index of element=w225:i32)  [unwired: 1 in]
          n88 = Greater Or Equal To 0?(x=w225) -> (x >= 0?=w226:bool)
          n89 = case shown="True" w226 {
            tunnel: w231 -> [w239 w243]
            tunnel: [w239 w242] -> w230
            tunnel: [_ w241] -> w229
            frame False {
            }
            frame True {
              n90 = call "Set IsConfigured.vi"("IsConfigured?"=FALSE, "SMO"=w243) -> ("error out"=w241:errorcluster, "SMO out"=w242:refnum<class "Instrument.lvclass">)  [unwired: 8 in]
            }
          }
          n91 = Scan From String(input string=w227, default 1=Instrument_Types--enum."DAQ" ("Type")) -> (output 1=w234:T8)  [unwired: 3 in, 3 out]
          n92 = call "Cast Instrument to Instrument Type.vi"("error in (no error)"=w229, "Type"=w234, "Instrument in"=w230, "Instrument Classes"=w238) -> ("error out"=w236:errorcluster, "Instrument Classes out"=w237:T13)  [unwired: 5 in, 1 out]
        }
        n93 = Bundle By Name(cluster=w221, "Instruments"=w212) -> (w222:T14)
        n94 = Merge Errors(w215, w217) -> (w214:errorcluster)
        n95 = call <vilib>:"Add State(s) to Queue__jki_lib_state_machine.vi"("State(s) in (\"\")"=w224) -> ("States Out"=w223:string)  [unwired: 14 in]
      }
      frame "Data: Open Instruments" {
        # "Do not put any code in this frame.\n(It is a separator no-op. You can make a copy of this frame to create a new Data frame)"
        n96 = Unbundle By Name(w252) -> ("Instruments"=w246:T13)
        n97 = call <vilib>:"Get Cluster Information.vi"("variant"=w246) -> ("error out"=w247:errorcluster, "cluster elements"=w248:variant[])  [unwired: 9 in]
        n98 = Cluster To Array(cluster=w246) -> (array=w249:refnum<class "Instrument.lvclass">[])
        n99 = for {
          tunnel: w249 -> [w259] mode=indexing
          tunnel: [w265] -> w244 mode=indexing
          shift-right: [w268] -> w245
          shift-left: w246 -> [w269]
          tunnel: w248 -> [w262] mode=indexing
          tunnel: w247 -> [w260]
          n100 = call <vilib>:"Get Type Information.vi"("error in (no error)"=w260, "variant"=w262) -> ("name"=w261:string)  [unwired: 5 in, 4 out]
          n101 = call "Get IsConfigured.vi"("SMO"=w259) -> ("error out"=w256:errorcluster, "IsConfigured?"=w257:bool, "SMO out"=w258:refnum<class "Instrument.lvclass">)  [unwired: 8 in]
          n102 = case shown="True" w257 {
            tunnel: [_ w274] -> w266
            tunnel: w258 -> [w270 w273]
            tunnel: [w270 w272] -> w267
            tunnel: w256 -> [_ w271]
            frame False {
            }
            frame True {
              n103 = call-dynamic "Open.vi"("error in (no error)"=w271, "Instrument in"=w273) -> ("error out"=w274:errorcluster, "Instrument out"=w272:refnum<class "Instrument.lvclass">)  [unwired: 8 in]
            }
          }
          n104 = Scan From String(input string=w261, default 1=Instrument_Types--enum."DAQ" ("Type")) -> (output 1=w263:T8)  [unwired: 3 in, 3 out]
          n105 = call "Cast Instrument to Instrument Type.vi"("error in (no error)"=w266, "Type"=w263, "Instrument in"=w267, "Instrument Classes"=w269) -> ("error out"=w265:errorcluster, "Instrument Classes out"=w268:T13)  [unwired: 5 in, 1 out]
        }
        n106 = Bundle By Name(cluster=w252, "Instruments"=w245) -> (w253:T14)
        n107 = Merge Errors(w250, w244) -> (w251:errorcluster)
        n108 = call <vilib>:"Add State(s) to Queue__jki_lib_state_machine.vi"("State(s) in (\"\")"=w255) -> ("States Out"=w254:string)  [unwired: 14 in]
      }
      frame "Data: Configure Magnet Type" {
        # "Do not put any code in this frame.\n(It is a separator no-op. You can make a copy of this frame to create a new Data frame)"
        n109 = Unbundle By Name(w275) -> ("Instruments.Magnet"=w280:refnum<class "Instrument.Cryostat.lvclass">)
        n110 = call <vilib>:"Get LV Class Name.vi"("error in (no error)"=w284, "object"=w280) -> ("error out"=w278:errorcluster, "class name"=w288:string)  [unwired: 8 in]
        n111 = Match Pattern(string=w288, regular expression="VRM") -> (offset past match=w286:i32)  [unwired: 1 in, 3 out]
        n112 = Greater Or Equal To 0?(x=w286) -> (x >= 0?=w276:bool)
        n113 = Select(t="Vector Magnet" ("new element/subarray"), s=w276, f="Magnet" ("element")) -> (s? t:f=w281:string)
        n114 = call "Set StateName.vi"("error in (no error)"=w278, "StateName"=w281, "SMO"=w280) -> ("error out"=w277:errorcluster, "SMO out"=w279:refnum<class "Instrument.Cryostat.lvclass">)  [unwired: 7 in]
        n115 = Bundle By Name(cluster=w275, "Instruments.Magnet"=w279) -> (w285:T14)
        n116 = call <vilib>:"Add State(s) to Queue__jki_lib_state_machine.vi"("State(s) in (\"\")"=w290) -> ("States Out"=w289:string)  [unwired: 14 in]
      }
      frame "Data: Close Instruments" {
        # "Data: Close Instruments\n(Close Instruments that are explicitly opened by this VI)"
        n117 = Unbundle By Name(w296) -> ("Instruments"=w293:T13)
        n118 = call <vilib>:"Get Cluster Information.vi"("variant"=w293) -> ("error out"=w291:errorcluster, "cluster elements"=w292:variant[])  [unwired: 9 in]
        n119 = Cluster To Array(cluster=w293) -> (array=w299:refnum<class "Instrument.lvclass">[])
        n120 = for {
          tunnel: w299 -> [w306] mode=indexing
          tunnel: [w312] -> w300 mode=indexing
          shift-right: [w315] -> w298
          shift-left: w293 -> [w316]
          tunnel: w292 -> [w309] mode=indexing
          tunnel: w291 -> [w307]
          n121 = call <vilib>:"Get Type Information.vi"("error in (no error)"=w307, "variant"=w309) -> ("name"=w308:string)  [unwired: 5 in, 4 out]
          n122 = call "Get IsConfigured.vi"("SMO"=w306) -> ("error out"=w303:errorcluster, "IsConfigured?"=w305:bool, "SMO out"=w304:refnum<class "Instrument.lvclass">)  [unwired: 8 in]
          n123 = case shown="True" w305 {
            tunnel: [w317 w321] -> w313
            tunnel: w304 -> [w318 w320]
            tunnel: [w318 w319] -> w314
            tunnel: w303 -> [w317 _]
            frame False {
            }
            frame True {
              n124 = call-dynamic "Close.vi"("Instrument in"=w320) -> ("error out"=w321:errorcluster, "Instrument out"=w319:refnum<class "Instrument.lvclass">)  [unwired: 9 in]
            }
          }
          n125 = Scan From String(input string=w308, default 1=Instrument_Types--enum."DAQ" ("Type")) -> (output 1=w310:T8)  [unwired: 3 in, 3 out]
          n126 = call "Cast Instrument to Instrument Type.vi"("error in (no error)"=w313, "Type"=w310, "Instrument in"=w314, "Instrument Classes"=w316) -> ("error out"=w312:errorcluster, "Instrument Classes out"=w315:T13)  [unwired: 5 in, 1 out]
        }
        n127 = Bundle By Name(cluster=w296, "Instruments"=w298) -> (w295:T14)
        n128 = Merge Errors(w297, w300) -> (w294:errorcluster)
        n129 = call <vilib>:"Add State(s) to Queue__jki_lib_state_machine.vi"("State(s) in (\"\")"=w302) -> ("States Out"=w301:string)  [unwired: 14 in]
      }
      frame "Data: UI Stop" {
        # "Data: UI Stop\n(Used to record when stop signal comes from UI (front panel stop or panel close)"
        n130 = Scan From String(input string=w324, default 1=FALSE) -> (output 1=w323:bool)  [unwired: 3 in, 3 out]
        n131 = Bundle By Name(cluster=w325, "UI stop"=w323) -> (w326:T14)
        n132 = call <vilib>:"Add State(s) to Queue__jki_lib_state_machine.vi"("State(s) in (\"\")"=w329) -> ("States Out"=w328:string)  [unwired: 14 in]
      }
      frame "Data: Cleanup" {
        # "Cleanup any data and references, here.\n(this is called automatically, by the Macro: Exit)"
        n133 = Unbundle By Name(w339) -> ("Transport"=w344:refnum<class "Transport.lvclass">, "Execution:State"=w336:T7, "C.E."=w335:refnum<class "Control Experiment.lvclass">, "Instruments"=w334:T13, "Core.Current VI Reference"=w342:refnum<vi>)
        n134 = case shown="\"Run top level\"" w336 {
          tunnel: [w350 w355] -> w333
          tunnel: w335 -> [w350 w354]
          tunnel: w331 -> [w348 w352]
          tunnel: [w348 w353] -> w330
          tunnel: w334 -> [w349 w351]
          tunnel: [w349 w351] -> w332
          frame Default {
          }
          frame "Run top level" {
            n135 = call "Close Dictionary.vi"("error in (no error)"=w352, "Control Experiment in"=w354) -> ("error out"=w353:errorcluster, "Control Experiment out"=w355:refnum<class "Control Experiment.lvclass">)  [unwired: 8 in]
          }
        }
        n136 = call "Write Instruments.vi"("error in (no error)"=w330, "Instruments"=w332, "Control Experiment in"=w333) -> ("error out"=w337:errorcluster, "Control Experiment out"=w338:refnum<class "Control Experiment.lvclass">)  [unwired: 7 in]
        n137 = call "Write Dependencies.vi"("error in (no error)"=w337, "Control Experiment"=w338, "Transport in"=w344) -> ("error out"=w341:errorcluster, "Transport out"=w345:refnum<class "Transport.lvclass">)  [unwired: 7 in]
        n138 = Bundle By Name(cluster=w339, "Transport"=w345) -> (w343:T14)
        n139 = Close Reference(reference=w342, error in (no error)=w341) -> (error out=w340:errorcluster)
        n140 = call <vilib>:"Add State(s) to Queue__jki_lib_state_machine.vi"("State(s) in (\"\")"=w347) -> ("States Out"=w346:string)  [unwired: 14 in]
      }
      frame "---------- UI ----------" {
        # "Do not put any code in this frame.\n(It is a separator no-op. You can make a copy of this frame to create a new UI frame)"
        n141 = call <vilib>:"Add State(s) to Queue__jki_lib_state_machine.vi"("State(s) in (\"\")"=w359) -> ("States Out"=w358:string)  [unwired: 14 in]
      }
      frame "UI: Initialize" {
        # "Initialize the User Interface, here.\n(this is called automatically, by the Macro: Init)"
        n142 = call <userlib>:"Tick Count (ms)__ogtk.vi"("error in (no error)"=w368) -> ("error out"=w367:errorcluster, "millisecond timer value"=w366:u32)  [unwired: 9 in]
        n143 = Unbundle By Name(w361) -> ("Run Time System?"=w360:bool)
        n144 = call <userlib>:"Fit VI window to Largest Dec__ogtk.vi"("error in (no error)"=w367, "border spacing (2 px)"=0) -> ("error out"=w363:errorcluster)  [unwired: 4 in, 1 out]
        n145 = local read "Emergency Stop Visible?"() -> (w362:bool)
        n146 = invoke on="stop" class="Bool (strict)" method="Reinit To Default"() -> ()  [unwired: 3 in, 3 out]
        n147 = property on="Emergency Stop Visible?" class="Bool (strict)"("Val(Sgnl)"=w362) -> ()  [unwired: 2 in, 2 out]
        n148 = property on="Start" class="Bool (strict)"("Visible"=w360) -> ()  [unwired: 2 in, 2 out]
        n149 = Bundle By Name(cluster=w361, "ms [0]"=w366, "ms [i]"=w366) -> (w364:T14)
        n150 = call <vilib>:"Add State(s) to Queue__jki_lib_state_machine.vi"("State(s) in (\"\")"=w370) -> ("States Out"=w369:string)  [unwired: 14 in]
      }
      frame "UI: Cursor Set" {
        # "Argument"
        # "Set and Unset Cursor Busy.\n(Usage: \"UI: Cursor Set >> Busy|Idle\")"
        n151 = case shown="\"Idle\", Default" w371 {
          tunnel: w373 -> [w378 w380]
          tunnel: [w377 w379] -> w372
          frame "Idle", Default {
            n152 = call <vilib>:"Unset Busy.vi"("error in (no error)"=w378) -> ("error out"=w377:errorcluster)  [unwired: 10 in]
          }
          frame "Busy" {
            n153 = call <vilib>:"Set Busy.vi"("error in (no error)"=w380) -> ("error out"=w379:errorcluster)  [unwired: 9 in, 1 out]
          }
        }
        n154 = call <vilib>:"Add State(s) to Queue__jki_lib_state_machine.vi"("State(s) in (\"\")"=w376) -> ("States Out"=w375:string)  [unwired: 14 in]
      }
      frame "UI: Emergency Stop Visible" {
        # "Do not put any code in this frame.\n(It is a separator no-op. You can make a copy of this frame to create a new UI frame)"
        n155 = Scan From String(input string=w383, default 1=FALSE) -> (output 1=w381:bool)  [unwired: 3 in, 3 out]
        n156 = property on="Emergency Stop 1" class="Bool"("Visible"=w381) -> ()  [unwired: 2 in, 2 out]
        n157 = property on="Emergency Stop 2" class="Bool"("Visible"=w381) -> ()  [unwired: 2 in, 2 out]
        n158 = property on="Emergency Stop 3" class="Bool"("Visible"=w381) -> ()  [unwired: 2 in, 2 out]
        n159 = property on="Emergency Stop 4" class="Bool"("Visible"=w381) -> ()  [unwired: 2 in, 2 out]
        n160 = call <vilib>:"Add State(s) to Queue__jki_lib_state_machine.vi"("State(s) in (\"\")"=w387) -> ("States Out"=w386:string)  [unwired: 14 in]
      }
      frame "UI: Update Timer" {
        n161 = Unbundle By Name(w399) -> ("ms [0]"=w400:u32)
        n162 = call <userlib>:"Tick Count (ms)__ogtk.vi"("error in (no error)"=w390) -> ("error out"=w389:errorcluster, "millisecond timer value"=w394:u32)  [unwired: 9 in]
        n163 = Subtract(x=w394, y=w400) -> (x-y=w397:u32)
        n164 = call <userlib>:"MGI Milliseconds Since Last Call.vi"("Error In"=w389) -> ("ms"=→"time b/w points (ms)":u32, "Error Out"=w395:errorcluster)  [unwired: 5 in]
        n165 = To Double Precision Float(number=w397) -> (double precision float=w393:dbl)
        n166 = To Double Precision Float(number=u32 1000 ("x")) -> (double precision float=w392:dbl)
        n167 = Bundle By Name(cluster=w399, "ms [i]"=w394) -> (w398:T14)
        n168 = Divide(x=w393, y=w392) -> (x/y=w401:dbl)
        n169 = To Long Integer(number=w401) -> (32bit integer=→"elapsed time (s)":i32)
        n170 = call <vilib>:"Add State(s) to Queue__jki_lib_state_machine.vi"("State(s) in (\"\")"=w403) -> ("States Out"=w402:string)  [unwired: 14 in]
      }
      frame "UI: Update Status" {
        # "Do not put any code in this frame.\n(It is a separator no-op. You can make a copy of this frame to create a new UI frame)"
        n171 = local read "Instrument Status"() -> (w406:string)
        n172 = To Lower Case(string=w405) -> (all lower case string=w413:string)
        n173 = Empty String/Path?(string/path=w406) -> (empty?=w404:bool)
        n174 = Equal?(x=w413, y="reset") -> (x = y?=w412:bool)
        n175 = Format Into String(format string="%s, %s", w406, w405) -> (resulting string=w408:string)  [unwired: 2 in, 1 out]
        n176 = Select(t=w405, s=w404, f=w408) -> (s? t:f=w407:string)
        n177 = Select(t="", s=w412, f=w407) -> (s? t:f=→"Instrument Status":string)
        n178 = call <vilib>:"Add State(s) to Queue__jki_lib_state_machine.vi"("State(s) in (\"\")"=w418) -> ("States Out"=w417:string)  [unwired: 14 in]
      }
      frame "UI: Update Graph Axis Labels" {
        w421 = "sweep (V)" ("string")
        n179 = control-ref of="AO"() -> (w423:refnum<vi>)
        n180 = control-ref of="AI"() -> (w422:refnum<vi>)
        n181 = control-ref of="2 Terminal"() -> (w427:refnum<vi>)
        n182 = control-ref of="4 Terminal"() -> (w426:refnum<vi>)
        n183 = control-ref of="Lockin (X)"() -> (w436:refnum<vi>)
        n184 = control-ref of="Lockin (Y)"() -> (w435:refnum<vi>)
        n185 = control-ref of="Resistance"() -> (w433:refnum<vi>)
        n186 = control-ref of="Conductance"() -> (w428:refnum<vi>)
        n187 = local read "Units"() -> (w431:enum16{"ohms & siemens", "h/e2 & e2/h"})
        n188 = case shown="\"h/e2 & e2/h\"" w431 {
          tunnel: ["R (ohms)" "R (h/e2)"] -> w430
          tunnel: ["G (siemens)" "G (e2/h)"] -> w429
          frame "ohms & siemens", Default {
          }
          frame "h/e2 & e2/h" {
          }
        }
        n189 = property on="Property Node" class="XYGraph (strict)"(reference=w427, "XScale.NameLbl.Text"=w421) -> (error out=w424:errorcluster)  [unwired: 1 in, 1 out]
        n190 = property on="Property Node" class="XYGraph (strict)"(reference=w426, "XScale.NameLbl.Text"=w421) -> (error out=w425:errorcluster)  [unwired: 1 in, 1 out]
        n191 = property on="Property Node" class="XYGraph (strict)"(reference=w436, "XScale.NameLbl.Text"=w421) -> (error out=w440:errorcluster)  [unwired: 1 in, 1 out]
        n192 = property on="Property Node" class="XYGraph (strict)"(reference=w435, "XScale.NameLbl.Text"=w421) -> (error out=w441:errorcluster)  [unwired: 1 in, 1 out]
        n193 = property on="Property Node" class="XYGraph (strict)"(reference=w433, "XScale.NameLbl.Text"=w421, "YScale.NameLbl.Text"=w430) -> (error out=w442:errorcluster)  [unwired: 1 in, 1 out]
        n194 = property on="Property Node" class="XYGraph (strict)"(reference=w428, "XScale.NameLbl.Text"=w421, "YScale.NameLbl.Text"=w429) -> (error out=w432:errorcluster)  [unwired: 1 in, 1 out]
        n195 = property on="Property Node" class="XYGraph (strict)"(reference=w423, "XScale.NameLbl.Text"=w421) -> (error out=w419:errorcluster)  [unwired: 1 in, 1 out]
        n196 = property on="Property Node" class="XYGraph (strict)"(reference=w422, "XScale.NameLbl.Text"=w421) -> (error out=w420:errorcluster)  [unwired: 1 in, 1 out]
        n197 = Merge Errors(w419, w420, w424, w425, w440, w441, w442, w432, w438) -> (w437:errorcluster)
        n198 = call <vilib>:"Clear Errors.vi"("error in (no error)"=w437) -> ("error out"=w439:errorcluster)  [unwired: 5 in, 1 out]
        n199 = call <vilib>:"Add State(s) to Queue__jki_lib_state_machine.vi"("State(s) in (\"\")"=w444) -> ("States Out"=w443:string)  [unwired: 14 in]
      }
      frame "UI: Update Lockin Graph Legend" {
        n200 = Unbundle By Name(w457) -> ("Results (Dictionary)"=w454:cluster{"key":string, "value":dbl}[])
        n201 = call <userlib>:"Parse Results (all).vi"("Type"=Results_Type--Enum."X", "error in (no error)"=w455, "Results (Dictionary)"=w454) -> ("error out"=w456:errorcluster, "Label"=w451:string[])  [unwired: 5 in, 2 out]
        n202 = Array Size(array=w451) -> (size(s)=w452:i32)
        n203 = for {
          tunnel: w456 -> [w469]
          tunnel: w451 -> [w465] mode=indexing
          tunnel: w452 -> [w464]
          tunnel: [w463] -> w450 mode=indexing
          tunnel: [w462] -> w449 mode=indexing
          i -> [w468]
          n204 = control-ref of="Lockin (X)"() -> (w466:refnum<vi>)
          n205 = property on="Property Node" class="XYGraph (strict)"(reference=w466, error in=w469, "Active Plot"=w468, "Plot.Plot Name"=w465, "LegPlotMin"=w464) -> (error out=w462:errorcluster)  [unwired: 1 out]
          n206 = control-ref of="Lockin (Y)"() -> (w467:refnum<vi>)
          n207 = property on="Property Node" class="XYGraph (strict)"(reference=w467, "Active Plot"=w468, "Plot.Plot Name"=w465, "LegPlotMin"=w464) -> (error out=w463:errorcluster)  [unwired: 1 in, 1 out]
        }
        n208 = Merge Errors(w450, w449) -> (w453:errorcluster)
        n209 = call <vilib>:"Clear Errors.vi"("error in (no error)"=w453) -> ("error out"=w459:errorcluster)  [unwired: 5 in, 1 out]
        n210 = call <vilib>:"Add State(s) to Queue__jki_lib_state_machine.vi"("State(s) in (\"\")"=w461) -> ("States Out"=w460:string)  [unwired: 14 in]
      }
      frame "UI: Update Wfm Graph Legend" {
        n211 = Unbundle By Name(w478) -> ("AO Waveforrm"=w475:waveform(dbl)[], "AI Waveform"=w474:waveform(dbl)[])
        n212 = Array Size(array=w474) -> (size(s)=w473:i32)
        n213 = Array Size(array=w475) -> (size(s)=w476:i32)
        n214 = for {
          N: w476 -> [w489]
          tunnel: [w494] -> w471 mode=indexing
          i -> [w493]
          n215 = Increment(x=w493) -> (x+1=w490:i32)
          n216 = control-ref of="AO"() -> (w495:refnum<vi>)
          n217 = Format Into String(format string="AO %d", w490) -> (resulting string=w491:string)  [unwired: 2 in, 1 out]
          n218 = property on="Property Node" class="XYGraph (strict)"(reference=w495, "Active Plot"=w493, "Plot.Plot Name"=w491, "LegPlotMin"=w489) -> (error out=w494:errorcluster)  [unwired: 1 in, 1 out]
        }
        n219 = for {
          N: w473 -> [w483]
          tunnel: [w488] -> w472 mode=indexing
          i -> [w487]
          n220 = Increment(x=w487) -> (x+1=w484:i32)
          n221 = control-ref of="AI"() -> (w482:refnum<vi>)
          n222 = Format Into String(format string="AI %d", w484) -> (resulting string=w485:string)  [unwired: 2 in, 1 out]
          n223 = property on="Property Node" class="XYGraph (strict)"(reference=w482, "Active Plot"=w487, "Plot.Plot Name"=w485, "LegPlotMin"=w483) -> (error out=w488:errorcluster)  [unwired: 1 in, 1 out]
        }
        n224 = Merge Errors(w471, w472, w470) -> (w477:errorcluster)
        n225 = call <vilib>:"Clear Errors.vi"("error in (no error)"=w477) -> ("error out"=w479:errorcluster)  [unwired: 5 in, 1 out]
        n226 = call <vilib>:"Add State(s) to Queue__jki_lib_state_machine.vi"("State(s) in (\"\")"=w481) -> ("States Out"=w480:string)  [unwired: 14 in]
      }
      frame "UI: Update R G Graph Legend" {
        n227 = local read "Resistance"() -> (w511:cluster{"X-array":dbl[], "Y-array":dbl[]}[])
        n228 = local read "Conductance"() -> (w512:cluster{"X-array":dbl[], "Y-array":dbl[]}[])
        n229 = Array Size(array=w511) -> (size(s)=w500:i32)
        n230 = Array Size(array=w512) -> (size(s)=w510:i32)
        n231 = Quotient & Remainder(x=w500, y=2) -> (floor(x/y)=w497:i32)  [unwired: 1 out]
        n232 = Quotient & Remainder(x=w510, y=2) -> (floor(x/y)=w504:i32)  [unwired: 1 out]
        n233 = Greater?(x=w497, y=1) -> (0:w496:bool)
        n234 = Greater?(x=w504, y=1) -> (0:w507:bool)
        n235 = case shown="False" w496 {
          tunnel: string[] ["R2T", "R4T"] -> [w520 w523]
          tunnel: [w520 w521] -> w499
          tunnel: w497 -> [_ w522]
          frame False {
          }
          frame True {
            n236 = for {
              N: w522 -> [_]
              tunnel: w523 -> [w526]
              tunnel: [w524] -> w521 mode=concatenating
              i -> [w528]
              n237 = call <vilib>:"Space Constant.vi"() -> ("String"=w527:string)
              n238 = Format Into String(initial string=w527, w528) -> (resulting string=w525:string)  [unwired: 2 in, 1 out]
              n239 = for {
                tunnel: w526 -> [w531] mode=indexing
                tunnel: w525 -> [w530]
                tunnel: [w529] -> w524 mode=indexing
                n240 = Concatenate Strings(w531, w530) -> (w529:string)
              }
            }
          }
        }
        n241 = case shown="False" w507 {
          tunnel: string[] ["G2T", "G4T"] -> [w532 w535]
          tunnel: [w532 w533] -> w508
          tunnel: w504 -> [_ w534]
          frame False {
          }
          frame True {
            n242 = for {
              N: w534 -> [_]
              tunnel: w535 -> [w538]
              tunnel: [w536] -> w533 mode=concatenating
              i -> [w540]
              n243 = call <vilib>:"Space Constant.vi"() -> ("String"=w539:string)
              n244 = Format Into String(initial string=w539, w540) -> (resulting string=w537:string)  [unwired: 2 in, 1 out]
              n245 = for {
                tunnel: w538 -> [w543] mode=indexing
                tunnel: w537 -> [w542]
                tunnel: [w541] -> w536 mode=indexing
                n246 = Concatenate Strings(w543, w542) -> (w541:string)
              }
            }
          }
        }
        n247 = for {
          N: w510 -> [w551]
          tunnel: [w552] -> w513 mode=indexing
          tunnel: w508 -> [w549] mode=indexing
          i -> [w550]
          n248 = control-ref of="Conductance"() -> (w553:refnum<vi>)
          n249 = property on="Property Node" class="XYGraph (strict)"(reference=w553, "Active Plot"=w550, "Plot.Plot Name"=w549, "LegPlotMin"=w551) -> (error out=w552:errorcluster)  [unwired: 1 in, 1 out]
        }
        n250 = for {
          N: w500 -> [w546]
          tunnel: [w548] -> w514 mode=indexing
          tunnel: w499 -> [w544] mode=indexing
          i -> [w547]
          n251 = control-ref of="Resistance"() -> (w545:refnum<vi>)
          n252 = property on="Property Node" class="XYGraph (strict)"(reference=w545, "Active Plot"=w547, "Plot.Plot Name"=w544, "LegPlotMin"=w546) -> (error out=w548:errorcluster)  [unwired: 1 in, 1 out]
        }
        n253 = Merge Errors(w513, w514, w503) -> (w515:errorcluster)
        n254 = call <vilib>:"Add State(s) to Queue__jki_lib_state_machine.vi"("State(s) in (\"\")"=w519) -> ("States Out"=w518:string)  [unwired: 14 in]
        n255 = call <vilib>:"Clear Errors.vi"("error in (no error)"=w515) -> ("error out"=w517:errorcluster)  [unwired: 5 in, 1 out]
      }
      frame "UI: Update AO AI Graphs" {
        n256 = Unbundle By Name(w566) -> ("Sweep Value"=w554:dbl, "AO Waveforrm"=w560:waveform(dbl)[], "AI Waveform"=w561:waveform(dbl)[])  [unwired: 1 out]
        n257 = To Lower Case(string=w562) -> (all lower case string=w563:string)
        n258 = Equal?(x=w563, y="reset") -> (x = y?=w557:bool)
        n259 = for {
          tunnel: w560 -> [w570] mode=indexing
          tunnel: [w569] -> w556 mode=indexing
          n260 = Unbundle By Name(w570) -> ("Y"=w571:dbl[])
          n261 = Index Array(array=w571) -> (element=w569:dbl)  [unwired: 1 in]
        }
        n262 = for {
          tunnel: w561 -> [w573] mode=indexing
          tunnel: [w572] -> w555 mode=indexing
          n263 = Unbundle By Name(w573) -> ("Y"=w574:dbl[])
          n264 = Index Array(array=w574) -> (element=w572:dbl)  [unwired: 1 in]
        }
        n265 = call "Graph Lockin vs Parameter.vi"("reset?"=w557, "Y"=w556, "X"=w554) -> ("Data vs Parameter"=→"AO":cluster{dbl[], dbl[]}[])  [unwired: 8 in]
        n266 = call "Graph Lockin vs Parameter.vi"("reset?"=w557, "Y"=w555, "X"=w554) -> ("Data vs Parameter"=→"AI":cluster{dbl[], dbl[]}[])  [unwired: 8 in]
        n267 = call <vilib>:"Add State(s) to Queue__jki_lib_state_machine.vi"("State(s) in (\"\")"=w568) -> ("States Out"=w567:string)  [unwired: 14 in]
      }
      frame "UI: Update Lockin Graphs" {
        # "results"
        n268 = Unbundle By Name(w585) -> ("Sweep Value"=w575:dbl, "Results (Dictionary)"=w591:cluster{"key":string, "value":dbl}[])  [unwired: 1 out]
        n269 = To Lower Case(string=w582) -> (all lower case string=w583:string)
        n270 = Equal?(x=w583, y="reset") -> (x = y?=w576:bool)
        n271 = call <userlib>:"Parse Results (all).vi"("Type"=Results_Type--Enum."X", "error in (no error)"=w580, "Results (Dictionary)"=w591) -> ("error out"=w587:errorcluster, "Data"=w578:dbl[], "Results (Dictionary)"=w588:cluster{"key":string, "value":dbl}[])  [unwired: 5 in, 1 out]
        n272 = call <userlib>:"Parse Results (all).vi"("Type"=Results_Type--Enum."Y", "error in (no error)"=w587, "Results (Dictionary)"=w588) -> ("error out"=w586:errorcluster, "Data"=w577:dbl[])  [unwired: 5 in, 2 out]
        n273 = call "Graph Lockin vs Parameter.vi"("reset?"=w576, "Y"=w578, "X"=w575) -> ("Data vs Parameter"=→"Lockin (X)":cluster{dbl[], dbl[]}[])  [unwired: 8 in]
        n274 = call "Graph Lockin vs Parameter.vi"("reset?"=w576, "Y"=w577, "X"=w575) -> ("Data vs Parameter"=→"Lockin (Y)":cluster{dbl[], dbl[]}[])  [unwired: 8 in]
        n275 = call <vilib>:"Add State(s) to Queue__jki_lib_state_machine.vi"("State(s) in (\"\")"=w593) -> ("States Out"=w592:string)  [unwired: 14 in]
      }
      frame "UI: Update R G Graphs" {
        # "Do not put any code in this frame.\n(It is a separator no-op. You can make a copy of this frame to create a new UI frame)"
        n276 = Unbundle By Name(w600) -> ("Amplitude"=w599:dbl[], "C.E."=w598:refnum<class "Control Experiment.lvclass">)
        n277 = call "Get Channel Indices.vi"("Control Experiment in"=w598) -> ("Indices"=w597:T16)  [unwired: 8 in, 2 out]
        n278 = local read "Lockin (Y)"() -> (w601:cluster{"Wavenumber":dbl[], "Data":dbl[]}[])
        n279 = local read "Lockin (X)"() -> (w602:cluster{"Wavenumber":dbl[], "Data":dbl[]}[])
        n280 = case shown="\"h/e2 & e2/h\"" "Units" {
          tunnel: [1.0 ("Siemens/(e2/h)") w610] -> w605
          frame "ohms & siemens", Default {
          }
          frame "h/e2 & e2/h" {
            w610 = 3.874046e-05  # Siemens/(e2/h)
          }
        }
        n281 = call "Graph R and G vs Parameter.vi"("indices"=w597, "AO Amp (V)"=w599, "Y vs Parameter"=w601, "X vs Parameter"=w602) -> ("G(Siemens) vs Parameter"=w604:cluster{"X-array":dbl[], dbl[]}[], "R(Ohms) vs Parameter"=w603:cluster{"X-array":dbl[], dbl[]}[])  [unwired: 6 in]
        n282 = call-poly <vilib>:"Multiply.vi"("y (1)"=w605, "XY-data"=w603) -> ("XY-data out"=→"Resistance":cluster{"X-array":dbl[], "Y-array":dbl[]}[])  [unwired: 8 in, 1 out]
        n283 = call-poly <vilib>:"Divide.vi"("y (1)"=w605, "XY-data"=w604) -> ("XY-data out"=→"Conductance":cluster{"X-array":dbl[], "Y-array":dbl[]}[])  [unwired: 8 in, 1 out]
        n284 = call <vilib>:"Add State(s) to Queue__jki_lib_state_machine.vi"("State(s) in (\"\")"=w608) -> ("States Out"=w607:string)  [unwired: 14 in]
      }
      frame "UI: Update Graphs from wfm" {
        # "Do not put any code in this frame.\n(It is a separator no-op. You can make a copy of this frame to create a new UI frame)"
        n285 = local read "Sweep Channels"() -> (w621:T2)
        n286 = Unbundle By Name(w623) -> ("Sweep_AO"=w618:waveform(dbl)[], "Sweep_AI"=w617:waveform(dbl)[], "Sweep_X"=w616:waveform(dbl)[], "Sweep_Y"=w615:waveform(dbl)[])  [unwired: 1 out]
        n287 = for {
          tunnel: [w639] -> w620
          tunnel: w621 -> [w642] mode=indexing
          stop <- w641 stop-if-true
          # "find the 1st enabled channel"
          n288 = Unbundle By Name(w642) -> ("Enable?"=w641:bool, "Channel"=w640:u16)
          n289 = Decrement(x=w640) -> (x-1=w639:u16)
        }
        n290 = Index Array(array=w618, index=w620) -> (element=w622:waveform(dbl))
        n291 = Unbundle By Name(w622) -> ("Y"=w614:dbl[])
        n292 = for {
          tunnel: w614 -> [w635]
          tunnel: w617 -> [w637] mode=indexing
          tunnel: [w636] -> w611 mode=indexing
          n293 = Unbundle By Name(w637) -> ("Y"=w638:dbl[])
          n294 = call <vilib>:"Initialize.vi"("Y-array"=w638, "X-array"=w635) -> ("XY-data out"=w636:cluster{"X-array":dbl[], "Y-array":dbl[]})  [unwired: 8 in, 1 out]
        }
        n295 = for {
          tunnel: w614 -> [w643]
          tunnel: w618 -> [w645] mode=indexing
          tunnel: [w644] -> w619 mode=indexing
          n296 = Unbundle By Name(w645) -> ("Y"=w646:dbl[])
          n297 = call <vilib>:"Initialize.vi"("Y-array"=w646, "X-array"=w643) -> ("XY-data out"=w644:cluster{"X-array":dbl[], "Y-array":dbl[]})  [unwired: 8 in, 1 out]
        }
        n298 = for {
          tunnel: w614 -> [w627]
          tunnel: w615 -> [w629] mode=indexing
          tunnel: [w628] -> w613 mode=indexing
          n299 = Unbundle By Name(w629) -> ("Y"=w630:dbl[])
          n300 = call <vilib>:"Initialize.vi"("Y-array"=w630, "X-array"=w627) -> ("XY-data out"=w628:cluster{"X-array":dbl[], "Y-array":dbl[]})  [unwired: 8 in, 1 out]
        }
        n301 = for {
          tunnel: w614 -> [w631]
          tunnel: w616 -> [w633] mode=indexing
          tunnel: [w632] -> w612 mode=indexing
          n302 = Unbundle By Name(w633) -> ("Y"=w634:dbl[])
          n303 = call <vilib>:"Initialize.vi"("Y-array"=w634, "X-array"=w631) -> ("XY-data out"=w632:cluster{"X-array":dbl[], "Y-array":dbl[]})  [unwired: 8 in, 1 out]
        }
        n304 = local write "AO"(w619) -> ()
        n305 = local write "AI"(w611) -> ()
        n306 = local write "Lockin (X)"(w612) -> ()
        n307 = local write "Lockin (Y)"(w613) -> ()
        n308 = call <vilib>:"Add State(s) to Queue__jki_lib_state_machine.vi"("State(s) in (\"\")"=w626) -> ("States Out"=w625:string)  [unwired: 14 in]
      }
      frame "UI: Update IV Graphs" {
        # "Do not put any code in this frame.\n(It is a separator no-op. You can make a copy of this frame to create a new UI frame)"
        n309 = Unbundle By Name(w663) -> ("Sweep_AI"=w660:waveform(dbl)[], "Sweep_AO"=w659:waveform(dbl)[], "C.E."=w665:refnum<class "Control Experiment.lvclass">)
        n310 = call "Get Channel Indices.vi"("error in (no error)"=w655, "Control Experiment in"=w665) -> ("error out"=w654:errorcluster, "Indices"=w652:T16)  [unwired: 7 in, 1 out]
        n311 = Decrement(x=w652) -> (x-1=w651:T16)
        n312 = Unbundle By Name(w651) -> ("I-"=w666:i32, "V1+"=w664:i32, "V1-"=w650:i32, "I+"=w669:i32)
        n313 = Equal?(x=w664, y=w650) -> (x = y?=w648:bool)
        n314 = Index Array(array=w660, index #1=w666, index #2=w664, index #3=w650) -> (element #1=w653:waveform(dbl), element #2=w668:waveform(dbl), element #3=w649:waveform(dbl))
        n315 = Index Array(array=w659, index=w669) -> (element=w670:waveform(dbl))
        n316 = case shown="False" w648 {
          tunnel: w668 -> [w674 w678]
          tunnel: w649 -> [_ w677]
          tunnel: [w674 w676] -> w647
          tunnel: [_ w675] -> _
          frame True {
          }
          frame False {
            n317 = Subtract(1:w677, 2:w678) -> (0:w676:waveform(dbl), 3:w675:errorcluster)  [unwired: 1 in]
          }
        }
        n318 = Unbundle By Name(w653) -> ("Y"=w658:dbl[])
        n319 = Unbundle By Name(w647) -> ("Y"=w657:dbl[])
        n320 = Unbundle By Name(w670) -> ("Y"=w656:dbl[])
        n321 = Bundle("Y"=w657, "Y"=w658) -> (w667:cluster{"Y":dbl[], "Y":dbl[]})  [unwired: 1 in]
        n322 = Bundle("Y"=w656, "Y"=w658) -> (w671:cluster{"Y":dbl[], "Y":dbl[]})  [unwired: 1 in]
        n323 = Build Array(w667) -> (→"4 Terminal":cluster{"Y":dbl[], "Y":dbl[]}[])
        n324 = Build Array(w671) -> (→"2 Terminal":cluster{"Y":dbl[], "Y":dbl[]}[])
        n325 = call <vilib>:"Add State(s) to Queue__jki_lib_state_machine.vi"("State(s) in (\"\")"=w673) -> ("States Out"=w672:string)  [unwired: 14 in]
      }
      frame "UI: Front Panel State" {
        # "Argument"
        # "Set Front Panel Open or Closed\n(Usage: \"UI: Front Panel State >> Open|Close\")"
        n326 = Unbundle By Name(w681) -> ("Core.Current VI Reference"=w680:refnum<vi>)
        n327 = case shown="\"Maximize\", \"Maximized\"" w679 {
          tunnel: w683 -> [w691 w706 w717 w730 w743]
          tunnel: [w693 w707 w719 w732 w745] -> w682
          tunnel: w680 -> [w692 w704 w718 w731 w744]
          frame "Open", "Standard", Default {
            w686 = T5."Standard" ("State")
            n328 = property class="VI"(reference=w692, error in=w691) -> (reference out=w689:refnum<vi>, error out=w690:errorcluster, "FP.State"=w688:T5)
            n329 = Not Equal?(x=w688, y=w686) -> (x != y?=w687:bool)
            n330 = case shown="False" w687 {
              tunnel: [w697 w699] -> w693
              tunnel: w690 -> [w696 w699]
              tunnel: w689 -> [w695 _]
              tunnel: w686 -> [w694 _]
              frame True {
                n331 = invoke class="VI" method="FP.Open"(reference=w695, error in=w696, "Activate"=TRUE, "State"=w694) -> (error out=w697:errorcluster)  [unwired: 1 in, 4 out]
              }
              frame False {
              }
            }
          }
          frame "Close", "Closed" {
            n332 = property class="VI"(reference=w704, error in=w706) -> (reference out=w703:refnum<vi>, error out=w705:errorcluster, "FP.State"=w701:T5)
            n333 = Not Equal?(x=w701, y=T5."Closed" ("Front Panel Window:State")) -> (x != y?=w700:bool)
            n334 = case shown="True" w700 {
              tunnel: [w708 w711] -> w707
              tunnel: w705 -> [w708 w710]
              tunnel: w703 -> [_ w709]
              frame False {
              }
              frame True {
                n335 = invoke class="VI" method="FP.Close"(reference=w709, error in=w710) -> (error out=w711:errorcluster)  [unwired: 1 in, 2 out]
              }
            }
          }
          frame "Hidden", "Hide" {
            w712 = T5."Hidden" ("State")
            n336 = property class="VI"(reference=w718, error in=w717) -> (reference out=w715:refnum<vi>, error out=w716:errorcluster, "FP.State"=w714:T5)
            n337 = Not Equal?(x=w714, y=w712) -> (x != y?=w713:bool)
            n338 = case shown="True" w713 {
              tunnel: [w723 w724] -> w719
              tunnel: w716 -> [w722 w724]
              tunnel: w715 -> [w721 _]
              tunnel: w712 -> [w720 _]
              frame True {
                n339 = invoke class="VI" method="FP.Open"(reference=w721, error in=w722, "State"=w720) -> (error out=w723:errorcluster)  [unwired: 2 in, 4 out]
              }
              frame False {
              }
            }
          }
          frame "Minimize", "Minimized" {
            w725 = T5."Minimized" ("State")
            n340 = property class="VI"(reference=w731, error in=w730) -> (reference out=w728:refnum<vi>, error out=w729:errorcluster, "FP.State"=w727:T5)
            n341 = Not Equal?(x=w727, y=w725) -> (x != y?=w726:bool)
            n342 = case shown="True" w726 {
              tunnel: [w736 w737] -> w732
              tunnel: w729 -> [w735 w737]
              tunnel: w728 -> [w734 _]
              tunnel: w725 -> [w733 _]
              frame True {
                n343 = invoke class="VI" method="FP.Open"(reference=w734, error in=w735, "State"=w733) -> (error out=w736:errorcluster)  [unwired: 2 in, 4 out]
              }
              frame False {
              }
            }
          }
          frame "Maximize", "Maximized" {
            w738 = T5."Maximized" ("State")
            n344 = property class="VI"(reference=w744, error in=w743) -> (reference out=w741:refnum<vi>, error out=w742:errorcluster, "FP.State"=w740:T5)
            n345 = Not Equal?(x=w740, y=w738) -> (x != y?=w739:bool)
            n346 = case shown="True" w739 {
              tunnel: [w749 w750] -> w745
              tunnel: w742 -> [w748 w750]
              tunnel: w741 -> [w747 _]
              tunnel: w738 -> [w746 _]
              frame True {
                n347 = invoke class="VI" method="FP.Open"(reference=w747, error in=w748, "State"=w746) -> (error out=w749:errorcluster)  [unwired: 2 in, 4 out]
              }
              frame False {
              }
            }
          }
        }
        n348 = call <vilib>:"Add State(s) to Queue__jki_lib_state_machine.vi"("State(s) in (\"\")"=w685) -> ("States Out"=w684:string)  [unwired: 14 in]
      }
      frame "---------- Macro ----------" {
        # "Do not put any code in this frame.\n(It is a separator no-op. You can make a copy of this frame to create a new Macro frame)"
        n349 = call <vilib>:"Add State(s) to Queue__jki_lib_state_machine.vi"("State(s) in (\"\")"=w754) -> ("States Out"=w753:string)  [unwired: 14 in]
      }
      frame "Macro: Initialize" {
        # "Initialization Macro\n(This is called once, when the VI starts)"
        n350 = Unbundle By Name(w757) -> ("Run Time System?"=w756:bool)
        n351 = Select(t="", s=w756, f="Macro: Start Sweep") -> (s? t:f=w760:string)
        n352 = call <vilib>:"Add State(s) to Queue__jki_lib_state_machine.vi"("State(s) in Front (\"\")"="Data: Initialize\nInitialize Core Data\nUI: Initialize\nUI: Front Panel State >> Open\nData: Initialize Top Level\nMacro: Initialize Instruments", "State(s) at Back (\"\")"=w760) -> ("States Out"=w758:string)  [unwired: 13 in]
        n353 = call <vilib>:"Add State(s) to Queue__jki_lib_state_machine.vi"("State(s) in Front (\"\")"=w758, "State(s) in (\"\")"=w764) -> ("States Out"=w763:string)  [unwired: 13 in]
      }
      frame "Macro: Initialize Instruments" {
        # "Do not put any code in this frame.\n(It is a separator no-op. You can make a copy of this frame to create a new Macro frame)"
        n354 = call <vilib>:"Add State(s) to Queue__jki_lib_state_machine.vi"("State(s) in Front (\"\")"="Data: Initialize Instruments\nData: Disable Unsupported Instruments\nData: Open Instruments\nData: Configure Magnet Type" ("State(s) in Front (\"\")"), "State(s) in (\"\")"=w769) -> ("States Out"=w768:string)  [unwired: 13 in]
      }
      frame "Macro: Measure Instruments" {
        # "Do not put any code in this frame.\n(It is a separator no-op. You can make a copy of this frame to create a new Macro frame)"
        n355 = Unbundle By Name(w778) -> ("Instruments"=w777:T13)
        n356 = Cluster To Array(cluster=w777) -> (array=w776:refnum<class "Instrument.lvclass">[])
        n357 = for {
          tunnel: w776 -> [w787] mode=indexing
          tunnel: [w790] -> w774 mode=indexing if=w785
          tunnel: [w783] -> w772 mode=indexing
          n358 = call "Get IsConfigured.vi"("SMO"=w787) -> ("error out"=w784:errorcluster, "IsConfigured?"=w785:bool, "SMO out"=w786:refnum<class "Instrument.lvclass">)  [unwired: 8 in]
          n359 = call "Get StateName.vi"("error in (no error)"=w784, "SMO"=w786) -> ("error out"=w783:errorcluster, "StateName"=w788:string)  [unwired: 7 in, 1 out]
          n360 = Concatenate Strings("Measure: " ("string"), w788) -> (w790:string)
        }
        n361 = Merge Errors(w770, w772) -> (w771:errorcluster)
        n362 = call <vilib>:"1D String Array to Delimited String.vi"("delimiter"="\n", "string array"=w774) -> ("delimited string"=w773:string)  [unwired: 9 in]
        n363 = call <vilib>:"Add State(s) to Queue__jki_lib_state_machine.vi"("State(s) in Front (\"\")"="UI: Update Status >> reset" ("State(s) in Front (\"\")"), "State(s) at Back (\"\")"=w773) -> ("States Out"=w779:string)  [unwired: 13 in]
        n364 = call <vilib>:"Add State(s) to Queue__jki_lib_state_machine.vi"("State(s) in Front (\"\")"=w779, "State(s) in (\"\")"=w782) -> ("States Out"=w781:string)  [unwired: 13 in]
      }
      frame "Macro: Start Sweep" {
        # "Macro: Start Sweep\n()"
        n365 = call <vilib>:"Add State(s) to Queue__jki_lib_state_machine.vi"("State(s) in Front (\"\")"="Sweep: Initialize\nFile: Write JSON\nMeasure: Time\nMacro: Measure Instruments\nUI: Update AO AI Graphs >> reset\nUI: Update Lockin Graphs >> reset\nUI: Update R G Graphs\nUI: Update Lockin Graph Legend\nUI: Update Wfm Graph Legend\nUI: Update R G Graph Legend\nUI: Update Graph Axis Labels\nSweep: Start\nMeasure: DAQ\nUI: Update AO AI Graphs >> reset\nUI: Update Lockin Graphs >> reset\nUI: Update R G Graphs" ("State(s) in Front (\"\")"), "State(s) in (\"\")"=w795) -> ("States Out"=w794:string)  [unwired: 13 in]
      }
      frame "Macro: Sweep" {
        # "Template Separator\n(You can make a copy of, or modify, this frame)"
        n366 = call <vilib>:"Add State(s) to Queue__jki_lib_state_machine.vi"("State(s) in Front (\"\")"="Measure: Time\nMacro: Measure Instruments\nUI: Update AO AI Graphs\nUI: Update Lockin Graphs\nUI: Update R G Graphs\nUI: Update Timer" ("State(s) in Front (\"\")"), "State(s) in (\"\")"=w800) -> ("States Out"=w799:string)  [unwired: 13 in]
      }
      frame "Macro: Stop Sweep" {
        # "only \"return to start\"\nwhen stop button is pushed,\notherwise defer to sweep configuration"
        # "Macro: Stop Sweep\n(handle sweep finish: stop, save data, return to start)"
        n367 = Unbundle By Name(w804) -> ("UI stop"=w803:bool)
        n368 = local read "Return to Start"() -> (w801:bool)
        n369 = And(x=w803, y=w801) -> (x .and. y?=w802:bool)
        n370 = Select(t="", s=w802, f="//") -> (s? t:f=w807:string)
        n371 = Format Into String(format string="Sweep: Stop\nMeasure: DAQ Sweep\nUI: Update AO AI Graphs\nUI: Update IV Graphs\nUI: Update Graphs from wfm\nUI: Update R G Graphs\nFile: Save Lockin\n%sSweep: Return to Start" ("State(s) in Front (\"\")"), w807) -> (resulting string=w805:string)  [unwired: 2 in, 1 out]
        n372 = call <vilib>:"Add State(s) to Queue__jki_lib_state_machine.vi"("State(s) in Front (\"\")"=w805, "State(s) in (\"\")"=w812) -> ("States Out"=w811:string)  [unwired: 13 in]
      }
      frame "Macro: Exit" {
        # "Exit Macro\n(This is called once, when the VI exits)"
        n373 = Unbundle By Name(w820) -> ("Core.Close Panel on Exit?"=w819:bool)
        n374 = Select(t="UI: Front Panel State >> Close", s=w819, f="") -> (s? t:f=w816:string)
        n375 = call <vilib>:"Add State(s) to Queue__jki_lib_state_machine.vi"("State(s) in Front (\"\")"="Macro: Stop Sweep\nData: Close Instruments", "State(s) in (\"\")"=w816, "State(s) at Back (\"\")"="Data: Cleanup\nExit") -> ("States Out"=w815:string)  [unwired: 12 in]
        n376 = call <vilib>:"Add State(s) to Queue__jki_lib_state_machine.vi"("State(s) in Front (\"\")"=w815, "State(s) in (\"\")"=w823) -> ("States Out"=w822:string)  [unwired: 13 in]
      }
      frame "---------- Sweep ----------" {
        # "Do not put any code in this frame.\n(It is a separator no-op. You can make a copy of this frame to create a new Macro frame)"
        n377 = call <vilib>:"Add State(s) to Queue__jki_lib_state_machine.vi"("State(s) in (\"\")"=w827) -> ("States Out"=w826:string)  [unwired: 14 in]
      }
      frame "Sweep: Initialize" {
        # "If Running Top Level\nOR\nSweep Channels from Transport\nare empty, use FP controls"
        # "Do not put any code in this frame.\n(It is a separator no-op. You can make a copy of this frame to create a new Macro frame)"
        n378 = Unbundle By Name(w857) -> ("Instruments.DAQ"=w837:refnum<class "Instrument.LockinAPI.lvclass">, "Execution:State"=w844:T7, "Transport"=w841:refnum<class "Transport.lvclass">)
        n379 = Unbundle By Name(w841) -> ("Sweep Channels"=w838:T2)
        n380 = Equal?(x=T7."Run top level" ("Execution:State"), y=w844) -> (x = y?=w842:bool)
        n381 = Empty Array?(array=w838) -> (empty?=w840:bool)
        n382 = Or(x=w842, y=w840) -> (x .or. y?=w839:bool)
        n383 = case shown="False" w839 {
          tunnel: "Sweep Time (s)" -> [_ w874]
          tunnel: [w867 w874] -> w847
          tunnel: "Initial Wait (s)" -> [_ w873]
          tunnel: [w868 w873] -> w848
          tunnel: [w865 w871] -> w849
          tunnel: "Sweep Channels" -> [_ w872]
          tunnel: [w866 w872] -> w850
          tunnel: w841 -> [w869 _]
          tunnel: "Sweep Tables" -> [_ w870]
          tunnel: "Return to Start" -> [_ w871]
          tunnel: [w864 w870] -> w845
          frame False {
            n384 = Unbundle By Name(w869) -> ("Sweep Time (s)"=w867:dbl, "Initial Wait (s)"=w868:dbl, "Return to Start"=w865:bool, "Sweep Channels"=w866:T2, "Sweep Tables"=w864:cluster{"Ch":i32, "Table":dbl[]}[])
          }
          frame True {
          }
        }
        n385 = Bundle By Name(cluster=T10 {"Sweep Time (s)"=0.0, "Initial Wait (s)"=0.0, "Return to Start"=FALSE, "Channels"=[]} ("Configure Sweep"), "Sweep Time (s)"=w847, "Initial Wait (s)"=w848, "Return to Start"=w849, "Channels"=w850) -> (w855:T10)
        n386 = for {
          tunnel: [w862] -> w833 mode=indexing
          tunnel: [w861] -> w831 mode=indexing
          tunnel: w845 -> [w863] mode=indexing
          n387 = Unbundle By Name(w863) -> ("Ch"=w862:i32, "Table"=w861:dbl[])
        }
        n388 = local write "Sweep Time (s)"(w847) -> ()
        n389 = local write "Initial Wait (s)"(w848) -> ()
        n390 = local write "Return to Start"(w849) -> ()
        n391 = local write "Sweep Channels"(w850) -> ()
        n392 = local write "Sweep Tables"(w845) -> ()
        n393 = call "Cast Lockin tsc.vi"("error in (no error)"=w834, "Instrument.LockinAPI in"=w837) -> ("error out"=w835:errorcluster, "Instrument.Lockin out"=w836:refnum<class "Instrument.Lockin.lvclass">)  [unwired: 8 in]
        n394 = call-dynamic "setSweep.vi"("error in (no error)"=w835, "Configure Sweep"=w855, "Instrument.Lockin in"=w836) -> ("error out"=w829:errorcluster, "Instrument.Lockin out"=w832:refnum<class "Instrument.Lockin.lvclass">)  [unwired: 7 in]
        n395 = call "setSweepTable.vim"("error in (no error)"=w829, "Table"=w831, "Channel"=w833, "Instrument.Lockin in"=w832) -> ("error out"=w828:errorcluster, "Instrument.Lockin out"=w830:refnum<class "Instrument.Lockin.lvclass">)  [unwired: 6 in]
        n396 = Bundle By Name(cluster=w857, "Instruments.DAQ"=w830) -> (w858:T14)
        n397 = call <vilib>:"Add State(s) to Queue__jki_lib_state_machine.vi"("State(s) in (\"\")"=w860) -> ("States Out"=w859:string)  [unwired: 14 in]
      }
      frame "Sweep: Start" {
        # "wait for sweeping to start"
        # "Do not put any code in this frame.\n(It is a separator no-op. You can make a copy of this frame to create a new Macro frame)"
        n398 = Unbundle By Name(w884) -> ("Instruments.DAQ"=w878:refnum<class "Instrument.LockinAPI.lvclass">)
        n399 = call "Cast Lockin tsc.vi"("error in (no error)"=w875, "Instrument.LockinAPI in"=w878) -> ("error out"=w876:errorcluster, "Instrument.Lockin out"=w877:refnum<class "Instrument.Lockin.lvclass">)  [unwired: 8 in]
        n400 = call-dynamic "startSweep.vi"("error in (no error)"=w876, "Instrument.Lockin in"=w877) -> ("error out"=w882:errorcluster, "Instrument.Lockin out"=w881:refnum<class "Instrument.Lockin.lvclass">)  [unwired: 8 in]
        n401 = call-dynamic "waitStatusSweepingStarted.vi"("error in (no error)"=w882, "Instrument.Lockin in"=w881) -> ("error out"=w879:errorcluster, "Instrument.Lockin out"=w880:refnum<class "Instrument.Lockin.lvclass">)  [unwired: 8 in]
        n402 = Bundle By Name(cluster=w884, "Instruments.DAQ"=w880) -> (w883:T14)
        n403 = call <vilib>:"Add State(s) to Queue__jki_lib_state_machine.vi"("State(s) in (\"\")"=w886) -> ("States Out"=w885:string)  [unwired: 14 in]
      }
      frame "Sweep: Check State" {
        # "Sweep: Check State\n(It is a separator no-op. You can make a copy of this frame to create a new Macro frame)"
        n404 = Unbundle By Name(w892) -> ("Instruments.DAQ"=w890:refnum<class "Instrument.LockinAPI.lvclass">)
        n405 = call "Cast Lockin tsc.vi"("error in (no error)"=w887, "Instrument.LockinAPI in"=w890) -> ("error out"=w888:errorcluster, "Instrument.Lockin out"=w889:refnum<class "Instrument.Lockin.lvclass">)  [unwired: 8 in]
        n406 = call-dynamic "getStatus.vi"("error in (no error)"=w888, "Instrument.Lockin"=w889) -> ("error out"=w896:errorcluster, "state"=w895:T17, "Instrument.Lockin"=w891:refnum<class "Instrument.Lockin.lvclass">)  [unwired: 7 in]
        n407 = case shown="\"sweeping\"" w895 {
          tunnel: ["Macro: Exit" ("State(s) in Front (\"\")") "Macro: Sweep" ("State(s) in Front (\"\")")] -> w894
          frame Default {
          }
          frame "sweeping" {
          }
        }
        n408 = Bundle By Name(cluster=w892, "Instruments.DAQ"=w891) -> (w893:T14)
        n409 = call <vilib>:"Add State(s) to Queue__jki_lib_state_machine.vi"("State(s) in Front (\"\")"=w894, "State(s) in (\"\")"=w898) -> ("States Out"=w897:string)  [unwired: 13 in]
      }
      frame "Sweep: Stop" {
        # "Sweep: Stop\n(It is a separator no-op. You can make a copy of this frame to create a new Macro frame)"
        n410 = Unbundle By Name(w910) -> ("Instruments.DAQ"=w904:refnum<class "Instrument.LockinAPI.lvclass">)
        n411 = call "Cast Lockin tsc.vi"("error in (no error)"=w901, "Instrument.LockinAPI in"=w904) -> ("error out"=w902:errorcluster, "Instrument.Lockin out"=w903:refnum<class "Instrument.Lockin.lvclass">)  [unwired: 8 in]
        n412 = call-dynamic "stopSweep.vi"("error in (no error)"=w902, "Instrument.Lockin in"=w903) -> ("error out"=w908:errorcluster, "Instrument.Lockin out"=w907:refnum<class "Instrument.Lockin.lvclass">)  [unwired: 8 in]
        n413 = call-dynamic "waitStatusSweepingStopped.vi"("error in (no error)"=w908, "Instrument.Lockin in"=w907) -> ("error out"=w905:errorcluster, "Instrument.Lockin out"=w906:refnum<class "Instrument.Lockin.lvclass">)  [unwired: 8 in]
        n414 = Bundle By Name(cluster=w910, "Instruments.DAQ"=w906) -> (w909:T14)
        n415 = call <vilib>:"Add State(s) to Queue__jki_lib_state_machine.vi"("State(s) in (\"\")"=w912) -> ("States Out"=w911:string)  [unwired: 14 in]
      }
      frame "Sweep: Return to Start" {
        # "Sweep: Stop\n(It is a separator no-op. You can make a copy of this frame to create a new Macro frame)"
        n416 = local read "Sweep Channels"() -> (w932:T2)
        n417 = Unbundle By Name(w934) -> ("Instruments.DAQ"=w916:refnum<class "Instrument.LockinAPI.lvclass">)
        n418 = call "Cast Lockin tsc.vi"("error in (no error)"=w913, "Instrument.LockinAPI in"=w916) -> ("error out"=w914:errorcluster, "Instrument.Lockin out"=w915:refnum<class "Instrument.Lockin.lvclass">)  [unwired: 8 in]
        n419 = call-dynamic "getAOconfig.vi"("error in (no error)"=w914, "Instrument.Lockin in"=w915) -> ("error out"=w922:errorcluster, "AOconfig"=w931:T18, "Instrument.Lockin out"=w925:refnum<class "Instrument.Lockin.lvclass">)  [unwired: 7 in]
        n420 = for {
          tunnel: w932 -> [w942] mode=indexing
          tunnel: w931 -> [w944]
          tunnel: [w939] -> w926 mode=indexing
          n421 = Unbundle By Name(w942) -> ("Channel"=w941:u16, "Start"=w940:dbl)
          n422 = Decrement(x=w941) -> (x-1=w945:u16)
          n423 = Index Array(array=w944, index=w945) -> (element=w943:T19)
          n424 = Unbundle By Name(w943) -> ("Offset"=w938:dbl)
          n425 = Bundle By Name(cluster=w942, "Start"=w938, "End"=w940, "Pattern"=Sweep.Pattern--Enum."Smooth Ramp _/") -> (w939:T3)
        }
        n426 = Bundle By Name(cluster=T10 {"Sweep Time (s)"=0.0, "Initial Wait (s)"=0.0, "Return to Start"=FALSE, "Channels"=[]} ("Configure Sweep"), "Sweep Time (s)"=2.0, "Channels"=w926) -> (w927:T10)
        n427 = call-dynamic "setSweep.vi"("error in (no error)"=w922, "Configure Sweep"=w927, "Instrument.Lockin in"=w925) -> ("error out"=w929:errorcluster, "Instrument.Lockin out"=w930:refnum<class "Instrument.Lockin.lvclass">)  [unwired: 7 in]
        n428 = call-dynamic "startSweep.vi"("error in (no error)"=w929, "Instrument.Lockin in"=w930) -> ("error out"=w921:errorcluster, "Instrument.Lockin out"=w920:refnum<class "Instrument.Lockin.lvclass">)  [unwired: 8 in]
        n429 = call-dynamic "waitStatusSweepingStarted.vi"("error in (no error)"=w921, "Instrument.Lockin in"=w920) -> ("error out"=w918:errorcluster, "Instrument.Lockin out"=w919:refnum<class "Instrument.Lockin.lvclass">)  [unwired: 8 in]
        n430 = call-dynamic "waitStatusSweepingStopped.vi"("error in (no error)"=w918, "Instrument.Lockin in"=w919) -> ("error out"=w923:errorcluster, "Instrument.Lockin out"=w924:refnum<class "Instrument.Lockin.lvclass">)  [unwired: 8 in]
        n431 = Bundle By Name(cluster=w934, "Instruments.DAQ"=w924) -> (w933:T14)
        n432 = call <vilib>:"Add State(s) to Queue__jki_lib_state_machine.vi"("State(s) in (\"\")"=w936) -> ("States Out"=w935:string)  [unwired: 14 in]
      }
      frame "---------- Configure ----------" {
        # "Do not put any code in this frame.\n(It is a separator no-op. You can make a copy of this frame to create a new Macro frame)"
        n433 = call <vilib>:"Add State(s) to Queue__jki_lib_state_machine.vi"("State(s) in (\"\")"=w949) -> ("States Out"=w948:string)  [unwired: 14 in]
      }
      frame "Configure: Wait" {
        # "Do not put any code in this frame.\n(It is a separator no-op. You can make a copy of this frame to create a new Macro frame)"
        n434 = call <vilib>:"Add State(s) to Queue__jki_lib_state_machine.vi"("State(s) in (\"\")"=w953) -> ("States Out"=w952:string)  [unwired: 14 in]
      }
      frame "---------- Measure ----------" {
        # "Template Separator\n(You can make a copy of, or modify, this frame)"
        n435 = call <vilib>:"Add State(s) to Queue__jki_lib_state_machine.vi"("State(s) in (\"\")"=w957) -> ("States Out"=w956:string)  [unwired: 14 in]
      }
      frame "Measure: Time" {
        # "Measure: Time.\n()"
        n436 = Unbundle By Name(w961) -> ("C.E."=w963:refnum<class "Control Experiment.lvclass">)
        n437 = Get Date/Time In Seconds() -> (seconds since 1Jan1904=w966:timestamp)
        n438 = To Double Precision Float(number=w966) -> (double precision float=w958:dbl)
        n439 = call "Write Dictionary Element.vi"("error in (no error)"=w960, "value"=w958, "key"="Time", "Control Experiment in"=w963) -> ("error out"=w959:errorcluster, "Control Experiment out"=w964:refnum<class "Control Experiment.lvclass">)  [unwired: 6 in]
        n440 = Bundle By Name(cluster=w961, "C.E."=w964, "Time"=w958) -> (w965:T14)
        n441 = call <vilib>:"Add State(s) to Queue__jki_lib_state_machine.vi"("State(s) in (\"\")"=w968) -> ("States Out"=w967:string)  [unwired: 14 in]
      }
      frame "Measure: Temperature" {
        # "Measure: Temperature.\n(called dynamically if instrument is configured in Control Experiment.vi)"
        n442 = Unbundle By Name(w977) -> ("Instruments.Temperature"=w975:refnum<class "Instrument.Cryostat.lvclass">, "C.E."=w979:refnum<class "Control Experiment.lvclass">)
        n443 = call-dynamic "getTemperature.vi"("error in (no error)"=w981, "Instrument.Cryostat in"=w975) -> ("error out"=w974:errorcluster, "Temperature (K)"=w970:dbl, "Instrument.Cryostat out"=w978:refnum<class "Instrument.Cryostat.lvclass">)  [unwired: 5 in, 2 out]
        n444 = call "Write Dictionary Element.vi"("error in (no error)"=w974, "value"=w970, "key"="Temperature", "Control Experiment in"=w979) -> ("error out"=w972:errorcluster, "Control Experiment out"=w976:refnum<class "Control Experiment.lvclass">)  [unwired: 6 in]
        n445 = case shown="No Error" w972 {
          selector: w972 -> [w984 w990]
          tunnel: w970 -> [w988 _]
          tunnel: [w985 _] -> w969
          tunnel: [w984 w990] -> w971
          frame No Error {
            n446 = Format Into String(format string="T = %2f K", w988) -> (resulting string=w986:string)  [unwired: 2 in, 1 out]
            n447 = call <vilib>:"Build State String with Arguments__JKI_lib_State_Machine.vi"("Arguments (\"\")"=w986, "State"="UI: Update Status" ("format string")) -> ("State with Arguments"=w985:string)  [unwired: 4 in]
          }
          frame Error {
          }
        }
        n448 = Bundle By Name(cluster=w977, "Instruments.Temperature"=w978, "C.E."=w976, "Temperature"=w970) -> (w980:T14)
        n449 = call <vilib>:"Add State(s) to Queue__jki_lib_state_machine.vi"("State(s) in Front (\"\")"=w969, "State(s) in (\"\")"=w983) -> ("States Out"=w982:string)  [unwired: 13 in]
      }
      frame "Measure: Magnet" {
        # "Measure: Magnet.\n(called dynamically by if instrument is configured in Control Experiment.vi)"
        n450 = Unbundle By Name(w998) -> ("Instruments.Magnet"=w997:refnum<class "Instrument.Cryostat.lvclass">, "C.E."=w1001:refnum<class "Control Experiment.lvclass">)
        n451 = call-dynamic "getMagnet.vi"("error in (no error)"=w1000, "Instrument.Cryostat in"=w997) -> ("error out"=w996:errorcluster, "B Field (T)"=w992:dbl, "Instrument.Cryostat out"=w999:refnum<class "Instrument.Cryostat.lvclass">)  [unwired: 5 in, 2 out]
        n452 = call "Write Dictionary Element.vi"("error in (no error)"=w996, "value"=w992, "key"="Magnet", "Control Experiment in"=w1001) -> ("error out"=w994:errorcluster, "Control Experiment out"=w1002:refnum<class "Control Experiment.lvclass">)  [unwired: 6 in]
        n453 = case shown="No Error" w994 {
          selector: w994 -> [w1006 w1012]
          tunnel: w992 -> [w1010 _]
          tunnel: [w1007 _] -> w991
          tunnel: [w1006 w1012] -> w993
          frame No Error {
            n454 = Format Into String(format string="B = %2f T", w1010) -> (resulting string=w1008:string)  [unwired: 2 in, 1 out]
            n455 = call <vilib>:"Build State String with Arguments__JKI_lib_State_Machine.vi"("Arguments (\"\")"=w1008, "State"="UI: Update Status" ("format string")) -> ("State with Arguments"=w1007:string)  [unwired: 4 in]
          }
          frame Error {
          }
        }
        n456 = Bundle By Name(cluster=w998, "Instruments.Magnet"=w999, "C.E."=w1002, "Magnet"=w992) -> (w1003:T14)
        n457 = call <vilib>:"Add State(s) to Queue__jki_lib_state_machine.vi"("State(s) in Front (\"\")"=w991, "State(s) in (\"\")"=w1005) -> ("States Out"=w1004:string)  [unwired: 13 in]
      }
      frame "Measure: Vector Magnet" {
        # "Measure: Vector Magnet.\n(called dynamically by if instrument is configured in Control Experiment.vi)"
        n458 = Unbundle By Name(w1024) -> ("Instruments.Magnet"=w1021:refnum<class "Instrument.Cryostat.lvclass">, "C.E."=w1031:refnum<class "Control Experiment.lvclass">)
        n459 = case shown="\"X\"" Magnet_Axis--Enum."Z" ("Axis") {
          tunnel: [2 ("index") 0 ("index") 1 ("index")] -> w1026
          frame "Z", Default {
          }
          frame "X" {
          }
          frame "Y" {
          }
        }
        n460 = call-dynamic "getMagnetVector.vi"("error in (no error)"=w1020, "Instrument.Cryostat in"=w1021) -> ("error out"=w1015:errorcluster, "Field (T)"=w1017:dbl[], "Instrument.Cryostat out"=w1019:refnum<class "Instrument.Cryostat.lvclass">)  [unwired: 5 in, 2 out]
        n461 = for {
          tunnel: w1017 -> [w1037] mode=indexing
          tunnel: string[] ["Bx", "By", "Bz"] ("input 1") -> [w1036] mode=indexing
          shift-right: [w1038] -> w1030
          shift-left: w1031 -> [w1039]
          tunnel: w1015 -> [w1035]
          tunnel: [w1034] -> w1016
          n462 = call "Write Dictionary Element.vi"("error in (no error)"=w1035, "value"=w1037, "key"=w1036, "Control Experiment in"=w1039) -> ("error out"=w1034:errorcluster, "Control Experiment out"=w1038:refnum<class "Control Experiment.lvclass">)  [unwired: 6 in]
        }
        n463 = Index Array(array=w1017, index #4=w1026) -> (element #1=w1029:dbl, element #2=w1028:dbl, element #3=w1027:dbl, element #4=w1018:dbl)  [unwired: 3 in]
        n464 = case shown="No Error" w1016 {
          selector: w1016 -> [w1045 w1051]
          tunnel: w1029 -> [w1049 _]
          tunnel: [w1046 _] -> w1013
          tunnel: [w1045 w1051] -> w1022
          tunnel: w1028 -> [w1044 _]
          tunnel: w1027 -> [w1043 _]
          frame No Error {
            n465 = Format Into String(format string="B = [%2f, %2f, %2f]", w1049, w1044, w1043) -> (resulting string=w1047:string)  [unwired: 2 in, 1 out]
            n466 = call <vilib>:"Build State String with Arguments__JKI_lib_State_Machine.vi"("Arguments (\"\")"=w1047, "State"="UI: Update Status" ("format string")) -> ("State with Arguments"=w1046:string)  [unwired: 4 in]
          }
          frame Error {
          }
        }
        n467 = Bundle By Name(cluster=w1024, "Instruments.Magnet"=w1019, "C.E."=w1030, "Magnet"=w1018) -> (w1025:T14)
        n468 = call <vilib>:"Add State(s) to Queue__jki_lib_state_machine.vi"("State(s) in Front (\"\")"=w1013, "State(s) in (\"\")"=w1033) -> ("States Out"=w1032:string)  [unwired: 13 in]
      }
      frame "Measure: Capacitance" {
        # "Measure: Capacitance.\n(called dynamically if instrument is configured in Control Experiment.vi)"
        n469 = Unbundle By Name(w1060) -> ("Instruments.Capacitance"=w1059:refnum<class "Instrument.CBridge.lvclass">, "C.E."=w1062:refnum<class "Control Experiment.lvclass">)
        n470 = call-dynamic "getCapacitance.vi"("error in (no error)"=w1061, "Instrument.CBridge in"=w1059) -> ("error out"=w1056:errorcluster, "Capacitance (pF)"=w1055:dbl, "Instrument.CBridge out"=w1058:refnum<class "Instrument.CBridge.lvclass">)  [unwired: 7 in]
        n471 = call "Write Dictionary Element.vi"("error in (no error)"=w1056, "value"=w1055, "key"="Capacitance", "Control Experiment in"=w1062) -> ("error out"=w1054:errorcluster, "Control Experiment out"=w1063:refnum<class "Control Experiment.lvclass">)  [unwired: 6 in]
        n472 = case shown="No Error" w1054 {
          selector: w1054 -> [w1067 w1073]
          tunnel: w1055 -> [w1071 _]
          tunnel: [w1068 _] -> w1052
          tunnel: [w1067 w1073] -> w1053
          frame No Error {
            n473 = Format Into String(format string="C = %2f pF", w1071) -> (resulting string=w1069:string)  [unwired: 2 in, 1 out]
            n474 = call <vilib>:"Build State String with Arguments__JKI_lib_State_Machine.vi"("Arguments (\"\")"=w1069, "State"="UI: Update Status" ("format string")) -> ("State with Arguments"=w1068:string)  [unwired: 4 in]
          }
          frame Error {
          }
        }
        n475 = Bundle By Name(cluster=w1060, "Instruments.Capacitance"=w1058, "C.E."=w1063) -> (w1064:T14)
        n476 = call <vilib>:"Add State(s) to Queue__jki_lib_state_machine.vi"("State(s) in Front (\"\")"=w1052, "State(s) in (\"\")"=w1066) -> ("States Out"=w1065:string)  [unwired: 13 in]
      }
      frame "Measure: Strain Cell" {
        # "Measure: Strain Cell.\n(called dynamically if instrument is configured in Control Experiment.vi)"
        n477 = Unbundle By Name(w1082) -> ("Instruments.Strain Cell"=w1081:refnum<class "Instrument.Strain.lvclass">, "C.E."=w1084:refnum<class "Control Experiment.lvclass">)
        n478 = call-dynamic "getStrain.vi"("error in (no error)"=w1083, "Instrument.Strain in"=w1081) -> ("error out"=w1078:errorcluster, "Strain (V)"=w1074:dbl, "Instrument.Strain out"=w1080:refnum<class "Instrument.Strain.lvclass">)  [unwired: 7 in]
        n479 = call "Write Dictionary Element.vi"("error in (no error)"=w1078, "value"=w1074, "key"="Strain", "Control Experiment in"=w1084) -> ("error out"=w1077:errorcluster, "Control Experiment out"=w1085:refnum<class "Control Experiment.lvclass">)  [unwired: 6 in]
        n480 = case shown="No Error" w1077 {
          selector: w1077 -> [w1089 w1095]
          tunnel: w1074 -> [w1093 _]
          tunnel: [w1090 _] -> w1075
          tunnel: [w1089 w1095] -> w1076
          frame No Error {
            n481 = Format Into String(format string="Strain = %2f V", w1093) -> (resulting string=w1091:string)  [unwired: 2 in, 1 out]
            n482 = call <vilib>:"Build State String with Arguments__JKI_lib_State_Machine.vi"("Arguments (\"\")"=w1091, "State"="UI: Update Status" ("format string")) -> ("State with Arguments"=w1090:string)  [unwired: 4 in]
          }
          frame Error {
          }
        }
        n483 = Bundle By Name(cluster=w1082, "Instruments.Strain Cell"=w1080, "C.E."=w1085) -> (w1086:T14)
        n484 = call <vilib>:"Add State(s) to Queue__jki_lib_state_machine.vi"("State(s) in Front (\"\")"=w1075, "State(s) in (\"\")"=w1088) -> ("States Out"=w1087:string)  [unwired: 13 in]
      }
      frame "Measure: Delay Line" {
        # "Measure: Delay Line.\n(called dynamically if instrument is configured in Control Experiment.vi)"
        n485 = Unbundle By Name(w1104) -> ("Instruments.Delay Line"=w1103:refnum<class "Instrument.DelayLine.lvclass">, "C.E."=w1106:refnum<class "Control Experiment.lvclass">)
        n486 = call-dynamic "getDelay.vi"("error in (no error)"=w1105, "Instrument.DelayLine in"=w1103) -> ("error out"=w1100:errorcluster, "delay (ps)"=w1096:dbl, "Instrument.DelayLine out"=w1102:refnum<class "Instrument.DelayLine.lvclass">)  [unwired: 6 in, 1 out]
        n487 = call "Write Dictionary Element.vi"("error in (no error)"=w1100, "value"=w1096, "key"="Delay", "Control Experiment in"=w1106) -> ("error out"=w1099:errorcluster, "Control Experiment out"=w1107:refnum<class "Control Experiment.lvclass">)  [unwired: 6 in]
        n488 = case shown="No Error" w1099 {
          selector: w1099 -> [w1111 w1117]
          tunnel: w1096 -> [w1115 _]
          tunnel: [w1112 _] -> w1097
          tunnel: [w1111 w1117] -> w1098
          frame No Error {
            n489 = Format Into String(format string="Delay = %2f ps", w1115) -> (resulting string=w1113:string)  [unwired: 2 in, 1 out]
            n490 = call <vilib>:"Build State String with Arguments__JKI_lib_State_Machine.vi"("Arguments (\"\")"=w1113, "State"="UI: Update Status" ("format string")) -> ("State with Arguments"=w1112:string)  [unwired: 4 in]
          }
          frame Error {
          }
        }
        n491 = Bundle By Name(cluster=w1104, "Instruments.Delay Line"=w1102, "C.E."=w1107) -> (w1108:T14)
        n492 = call <vilib>:"Add State(s) to Queue__jki_lib_state_machine.vi"("State(s) in Front (\"\")"=w1097, "State(s) in (\"\")"=w1110) -> ("States Out"=w1109:string)  [unwired: 13 in]
      }
      frame "Measure: Rotator" {
        # "Measure: Delay Line.\n(called dynamically if instrument is configured in Control Experiment.vi)"
        n493 = Unbundle By Name(w1126) -> ("Instruments.Rotator"=w1125:refnum<class "Instrument.Cryostat.lvclass">, "C.E."=w1128:refnum<class "Control Experiment.lvclass">)
        n494 = call-dynamic "getAngle.vi"("error in (no error)"=w1127, "Instrument.Cryostat in"=w1125) -> ("error out"=w1122:errorcluster, "Angle (°)"=w1118:dbl, "Instrument.Cryostat out"=w1124:refnum<class "Instrument.Cryostat.lvclass">)  [unwired: 5 in, 2 out]
        n495 = call "Write Dictionary Element.vi"("error in (no error)"=w1122, "value"=w1118, "key"="Angle", "Control Experiment in"=w1128) -> ("error out"=w1121:errorcluster, "Control Experiment out"=w1129:refnum<class "Control Experiment.lvclass">)  [unwired: 6 in]
        n496 = case shown="No Error" w1121 {
          selector: w1121 -> [w1133 w1139]
          tunnel: w1118 -> [w1137 _]
          tunnel: [w1134 _] -> w1119
          tunnel: [w1133 w1139] -> w1120
          frame No Error {
            n497 = Format Into String(format string="Angle = %2f°", w1137) -> (resulting string=w1135:string)  [unwired: 2 in, 1 out]
            n498 = call <vilib>:"Build State String with Arguments__JKI_lib_State_Machine.vi"("Arguments (\"\")"=w1135, "State"="UI: Update Status" ("format string")) -> ("State with Arguments"=w1134:string)  [unwired: 4 in]
          }
          frame Error {
          }
        }
        n499 = Bundle By Name(cluster=w1126, "Instruments.Rotator"=w1124, "C.E."=w1129) -> (w1130:T14)
        n500 = call <vilib>:"Add State(s) to Queue__jki_lib_state_machine.vi"("State(s) in Front (\"\")"=w1119, "State(s) in (\"\")"=w1132) -> ("States Out"=w1131:string)  [unwired: 13 in]
      }
      frame "Measure: DAQ" {
        # "Gives the AI and AO waveform which refreshes as per the Lockin sampling parameters"
        # "Measure Lockin\n(Read intermediate values of the waveforms)"
        n501 = Unbundle By Name(w1156) -> ("Instruments.DAQ"=w1143:refnum<class "Instrument.LockinAPI.lvclass">)
        n502 = local read "Sweep Channels"() -> (w1146:T2)
        n503 = call "Cast Lockin tsc.vi"("error in (no error)"=w1140, "Instrument.LockinAPI in"=w1143) -> ("error out"=w1141:errorcluster, "Instrument.Lockin out"=w1142:refnum<class "Instrument.Lockin.lvclass">)  [unwired: 8 in]
        n504 = for {
          tunnel: [w1165] -> w1145
          tunnel: w1146 -> [w1168] mode=indexing
          stop <- w1167 stop-if-true
          # "find the 1st enabled channel"
          n505 = Unbundle By Name(w1168) -> ("Enable?"=w1167:bool, "Channel"=w1166:u16)
          n506 = Decrement(x=w1166) -> (x-1=w1165:u16)
        }
        n507 = call-dynamic "getAOconfig.vi"("error in (no error)"=w1141, "Instrument.Lockin in"=w1142) -> ("error out"=w1148:errorcluster, "AOconfig"=w1144:T18, "Instrument.Lockin out"=w1151:refnum<class "Instrument.Lockin.lvclass">)  [unwired: 7 in]
        n508 = call-dynamic "getAOwfm.vi"("error in (no error)"=w1148, "Instrument.Lockin in"=w1151) -> ("error out"=w1158:errorcluster, "AO Waveforrm"=w1152:waveform(dbl)[], "Instrument.Lockin out"=w1160:refnum<class "Instrument.Lockin.lvclass">)  [unwired: 7 in]
        n509 = call-dynamic "getAIwfm.vi"("error in (no error)"=w1158, "Instrument.Lockin in"=w1160) -> ("error out"=w1157:errorcluster, "AI Waveform"=w1153:waveform(dbl)[], "Instrument.Lockin out"=w1159:refnum<class "Instrument.Lockin.lvclass">)  [unwired: 7 in]
        n510 = Index Array(array=w1144, index=w1145) -> (element=w1150:T19)
        n511 = for {
          tunnel: [w1170] -> w1147 mode=indexing
          tunnel: w1144 -> [w1169] mode=indexing
          n512 = Unbundle By Name(w1169) -> ("Amplitude"=w1170:dbl)
        }
        n513 = call-dynamic "getResults.vi"("error in (no error)"=w1157, "Instrument.Lockin in"=w1159) -> ("error out"=w1162:errorcluster, "Results (Dictionary)"=w1161:cluster{"key":string, "value":dbl}[], "Instrument.Lockin out"=w1154:refnum<class "Instrument.Lockin.lvclass">)  [unwired: 6 in, 1 out]
        n514 = Unbundle By Name(w1150) -> ("Offset"=w1149:dbl)
        n515 = Bundle By Name(cluster=w1156, "Instruments.DAQ"=w1154, "Results (Dictionary)"=w1161, "AI Waveform"=w1153, "AO Waveforrm"=w1152, "Amplitude"=w1147, "Sweep Value"=w1149) -> (w1155:T14)
        n516 = call <vilib>:"Add State(s) to Queue__jki_lib_state_machine.vi"("State(s) in (\"\")"=w1164) -> ("States Out"=w1163:string)  [unwired: 14 in]
      }
      frame "Measure: DAQ Sweep" {
        # "Gives the AI and AO waveform which refreshes as per the Lockin sampling parameters"
        # "Measure: Lockin Sweep\n(get all sweep waveforms from lockin)"
        n517 = Unbundle By Name(w1183) -> ("Instruments.DAQ"=w1174:refnum<class "Instrument.LockinAPI.lvclass">)
        n518 = call "Cast Lockin tsc.vi"("error in (no error)"=w1171, "Instrument.LockinAPI in"=w1174) -> ("error out"=w1172:errorcluster, "Instrument.Lockin out"=w1173:refnum<class "Instrument.Lockin.lvclass">)  [unwired: 8 in]
        n519 = call-dynamic "getSweepData.vi"("error in (no error)"=w1172, "Instrument.Lockin in"=w1173) -> ("error out"=w1180:errorcluster, "SweepData"=w1175:T21, "Instrument.Lockin out"=w1181:refnum<class "Instrument.Lockin.lvclass">)  [unwired: 7 in]
        n520 = Unbundle By Name(w1175) -> ("AO"=w1179:waveform(dbl)[], "AI"=w1178:waveform(dbl)[], "X"=w1177:waveform(dbl)[], "Y"=w1176:waveform(dbl)[])
        n521 = Bundle By Name(cluster=w1183, "Instruments.DAQ"=w1181, "Sweep_AO"=w1179, "Sweep_AI"=w1178, "Sweep_X"=w1177, "Sweep_Y"=w1176) -> (w1182:T14)
        n522 = call <vilib>:"Add State(s) to Queue__jki_lib_state_machine.vi"("State(s) in (\"\")"=w1185) -> ("States Out"=w1184:string)  [unwired: 14 in]
      }
      frame "---------- File ----------" {
        # "Template Separator\n(You can make a copy of, or modify, this frame)"
        n523 = call <vilib>:"Add State(s) to Queue__jki_lib_state_machine.vi"("State(s) in (\"\")"=w1189) -> ("States Out"=w1188:string)  [unwired: 14 in]
      }
      frame "File: Configure" {
        # "Template Separator\n(You can make a copy of, or modify, this frame)"
        n524 = call <vilib>:"Add State(s) to Queue__jki_lib_state_machine.vi"("State(s) in (\"\")"=w1193) -> ("States Out"=w1192:string)  [unwired: 14 in]
      }
      frame "File: Write JSON" {
        # "Template Separator\n(You can make a copy of, or modify, this frame)"
        n525 = Unbundle By Name(w1201) -> ("C.E."=w1199:refnum<class "Control Experiment.lvclass">)
        n526 = call "Write JSON to Dictionary.vi"("error in (no error)"=w1196, "Control Experiment in"=w1199) -> ("error out"=w1197:errorcluster, "Control Experiment out"=w1198:refnum<class "Control Experiment.lvclass">)  [unwired: 8 in]
        n527 = local read "Sweep Time (s)"() -> (w1208:dbl)
        n528 = local read "Initial Wait (s)"() -> (w1209:dbl)
        n529 = local read "Return to Start"() -> (w1210:bool)
        n530 = local read "Sweep Channels"() -> (w1211:T2)
        n531 = local read "Sweep Tables"() -> (w1194:cluster{"Ch":i32, "Table":dbl[]}[])
        n532 = Bundle By Name(cluster=T12 {"Sweep Time (s)"=0.0, "Initial Wait (s)"=0.0, "Return to Start"=FALSE, "Sweep Channels"=[], "Sweep Tables"=[]} ("Lockin_Sweep"), "Sweep Time (s)"=w1208, "Initial Wait (s)"=w1209, "Return to Start"=w1210, "Sweep Channels"=w1211, "Sweep Tables"=w1194) -> (w1206:T12)
        n533 = call "To JSON Text.vim"("error in (no error)"=w1197, "Anything"=w1206) -> ("error out"=w1200:errorcluster, "<JSON>"=w1207:string)  [unwired: 8 in]
        n534 = call "Write Dictionary Element.vi"("error in (no error)"=w1200, "value"=w1207, "key"="<LockinSweep>", "Control Experiment in"=w1198) -> ("error out"=w1204:errorcluster, "Control Experiment out"=w1203:refnum<class "Control Experiment.lvclass">)  [unwired: 6 in]
        n535 = Bundle By Name(cluster=w1201, "C.E."=w1203) -> (w1202:T14)
        n536 = call <vilib>:"Add State(s) to Queue__jki_lib_state_machine.vi"("State(s) in (\"\")"=w1213) -> ("States Out"=w1212:string)  [unwired: 14 in]
      }
      frame "File: Save Lockin" {
        # "F --> create\nnew file\neach time\nthis state runs"
        # "build cluster array(s) of multiple 1D data, dynamically name waves"
        # "Template Separator\n(You can make a copy of, or modify, this frame)"
        n537 = Unbundle By Name(w1227) -> ("C.E."=w1230:refnum<class "Control Experiment.lvclass">, "Sweep_AO"=w1219:waveform(dbl)[], "Sweep_AI"=w1218:waveform(dbl)[], "Sweep_X"=w1217:waveform(dbl)[], "Sweep_Y"=w1221:waveform(dbl)[])
        n538 = Build Cluster Array(w1219, w1218, w1217, w1221) -> (w1214:cluster{"Sweep_Y":waveform(dbl)[]}[])
        n539 = for {
          shift-right: [w1237] -> w1222
          shift-left: w1220 -> [w1238]
          tunnel: string[] ["AO", "AI", "X", "Y"] -> [w1236] mode=indexing
          tunnel: [w1235] -> w1215 mode=concatenating
          tunnel: w1214 -> [w1234] mode=indexing
          n540 = Unbundle(w1234) -> ("Sweep_Y"=w1233:waveform(dbl)[])
          n541 = call "Data to Dictionary.vim"("Error in"=w1238, "Data in"=w1233, "Label in"=w1236) -> ("Error out"=w1237:errorcluster, "Data out"=w1235:T22[])  [unwired: 7 in]
        }
        n542 = call "Write Dictionary Elements (Loop).vi"("error in (no error)"=w1222, "Data in"=w1215, "Control Experiment in"=w1230) -> ("error out"=w1224:errorcluster, "Control Experiment out"=w1226:refnum<class "Control Experiment.lvclass">)  [unwired: 7 in]
        n543 = call "Save Transport TDMS File.vi"("append?"=FALSE, "error in (no error)"=w1224, "Control Experiment in"=w1226) -> ("error out"=w1225:errorcluster, "Control Experiment out"=w1229:refnum<class "Control Experiment.lvclass">)  [unwired: 7 in]
        n544 = Bundle By Name(cluster=w1227, "C.E."=w1229) -> (w1228:T14)
        n545 = call <vilib>:"Add State(s) to Queue__jki_lib_state_machine.vi"("State(s) in (\"\")"=w1232) -> ("States Out"=w1231:string)  [unwired: 14 in]
      }
    }
  }
  "error out" <- w2
  n546 = Unbundle By Name(w4) -> ("Transport"=→"Transport out":refnum<class "Transport.lvclass">)
